vi "BIAS_Client.vi"() -> ()   [LabVIEW 2012]
uses:
  <userlib>/bias2/subvis/ROI_rect.ctl
  <userlib>/bias2/subvis/Imaging_State.ctl
  <userlib>/bias2/subvis/Frame_Controls.ctl
  <userlib>/bias2/subvis/ui/CameraParameters.ctl
  <vilib>/Utility/error.llb/DialogType.ctl
  <userlib>/bias2/classes/CameraBase/CameraBase.lvclass
  <vilib>/event_ctls.llb/lveventtype.ctl
  <userlib>/bias2/subvis/zlock/ZLock.lvclass
  <userlib>/bias2/subvis/ExposureSettings.ctl
  <vilib>/addons/h5labview/H5F_mode.ctl
  <vilib>/Utility/file.llb/Read From Spreadsheet File (DBL).vi
  <vilib>/addons/h5labview/H5File.lvlib
  <vilib>/addons/h5labview/H5GroupObject.lvlib
  <vilib>/addons/h5labview/H5Attrib.lvlib
  <vilib>/addons/h5labview/H5Base.lvlib
  <vilib>/Analysis/NI_AALPro.lvlib
panel:
  in  "capture":T1 caption="Capture"
  in  "tools_zoom":T2 caption="Zoom tools"
  in  "tools_view":cluster{"sel":bool, "in":bool, "out":bool} caption="View tools"
  in  "files":T3 caption="Files"
  in  "stop":bool
  out "stop_time":dbl=11.582550000000003
  out "busy":bool caption="Busy"
  out "recent_error":bool caption="Error"
  out "remote":bool caption="Remote"
  out "acquiring":bool caption="Acquiring"
  out "img_OD":T4(plugin-control)
  out "image_raw":sgl[][](array[numeric])
  in  "tabs":T5(tab)=enum."Internal"
  in  "binning":cluster{"x":u8, "y":u8}={"x"=1, "y"=1}
  in  "effective_pixel":dbl caption="effective pixel size"
  in  "rotation":u16(ring) items=["Do not rotate", "Rotate 90°", "Rotate 180°", "Rotate -90°"]
  out "cam_params":cluster{"String":string, "value":variant}[](array[cluster])=[{"String"="TriggerSource", "value"=variant(string "Freerun")}, {"String"="Timeout", "value"=variant(u32 23583)}, {"String"="ShiftPixelBits", "value"=variant(bool FALSE)}, {"String"="PixelFormat", "value"=variant(string "Mono14")}] caption="Camera Parameters"
  in  "rois":T7(array[cluster])=[{"get"=FALSE, "set"=FALSE, "rect"={"left"=0, "top"=0, "right"=0, "bottom"=0}, "color"=16777224}, {"get"=FALSE, "set"=FALSE, "rect"={"left"=0, "top"=0, "right"=0, "bottom"=0}, "color"=6618880}, {"get"=FALSE, "set"=FALSE, "rect"={"left"=0, "top"=0, "right"=0, "bottom"=0}, "color"=16776960}, {"get"=FALSE, "set"=FALSE, "rect"={"left"=0, "top"=0, "right"=0, "bottom"=0}, "color"=4849919}]
  in  "camera name":string
  out "camera model":string="GX1920 (02-2410B), serial 0xF3101FDAB"
  in  "exposure":sgl=100.0 caption="exposure (ms)"
  out "location":string caption="camera location"
  out "roi_sensor":T6={"left"=0, "top"=0, "right"=1936, "bottom"=1456} caption="camera size"
  out "roi_capture":T6={"left"=686, "top"=399, "right"=1281, "bottom"=1004}
  out "keep":u8
  out "working dir":path
  out "current file":string
  in  "raw_ctrls":T8={"col_scheme"=0, "val_min"=100.0, "val_max"=16384.0, "automax"=FALSE} {"col_scheme" items=["Grayscale", "Rainbow", "Temperature", "-", "AlpineColors", "Amherst", "Aquamarine", "ArmyColors", "AtlanticColors", "AuroraColors", "AvocadoColors", "BeachColors", "BlueGreenYellow", "BrassTones", "BrightBands", "BrownCyanTones", "CandyColors", "CherryTones", "CMYKColors", "CoffeeTones", "DarkBands", "DarkRainbow", "DarkTerrain", "DeepSeaColors", "Default", "FallColors", "FruitPunchColors", "FuchsiaTones", "GrayTones", "GrayYellowTones", "GreenBrownTerrain", "GreenPinkTones", "IslandColors", "LabVIEW", "LakeColors", "LightTemperatureMap", "LightTerrain", "MintColors", "NeonColors", "NIST", "Pastel", "PearlColors", "PigeonTones", "PlumColors", "Rainbow", "RedBlueTones", "RedGreenSplit", "RoseColors", "RustTones", "SandyTerrain", "SiennaTones", "SolarColors", "SouthwestColors", "StarryNightColors", "SunsetColors", "TemperatureMap", "ThermometerColors", "ValentineTones", "WatermelonColors"]; "val_max" format="%_4g"; "val_min" format="%_4g"}
  in  "raw_list":i32(listbox)=-1 caption="Raw Frames"
  in  "hold_frames":bool caption="Hold last flat/dark frames"
  in  "histograms":bool caption="histogram"
  out "recent":string[](array[string]) caption="recent log messages"
  out "state":T9 caption="system state"
  in  "last error":T10={"status"=FALSE, "code"=42, "description"="", "time"=timestamp(3029490000.67111 s since 1904-01-01)} caption="most recent error:" {"time" format="%<%H:%M:%S %d/%m/%y>T"}
  in  "Parameters":T11={"name"="XY_1_Flea3", "sdk"="IMAQdx_Flea3_Firewire", "serial"=0, "port"=1024, "h5"=path "C:/Experiments/rb_chip/connectiontable.h5", "zlock server"="atomchip-1.nist.gov", "zlock port"=7339}
  out "sequencer":T12(array[cluster])
  out "roi_current":T6
  out "image_data":u16[][][](array[numeric])
  out "frame":i32=-1 caption="display_frame"
  out "BLACS port":u16
  out "image_size":i32[](array[numeric])
  out "attribs":variant[](array[variant])=[variant(i32 864), variant(i32 519), variant(i32 1176), variant(i32 878), variant(i64 0), variant(string "Freerun"), variant(u32 1), variant(u32 1), variant(i64 864), variant(i64 519), variant(i64 312), variant(i64 359), variant(dbl 100000.00149011612)]
  out "raw histograms":T13(array[cluster])
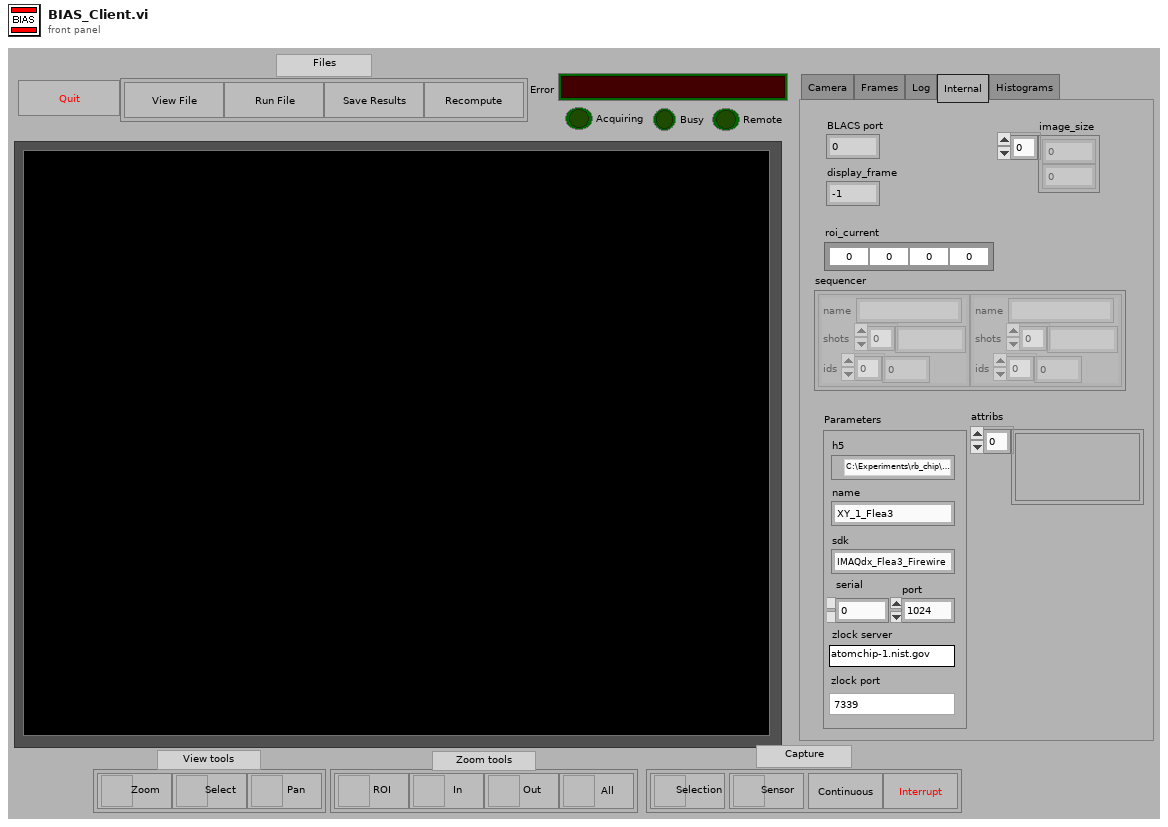
[diagram p1: front panel]
types:
  T1 = cluster{"roi":bool, "chip":bool, "continuous":bool, "abort":bool}
  T2 = cluster{"sel":bool, "in":bool, "out":bool, "all":bool}
  T3 = cluster{"open_file 2":bool, "open_file":bool, "save_file":bool, "open_file 3":bool}
  T4 = typedef "IMAQ Image.ctl" = refnum<image>
  T5 = enum32{"Camera", "Frames", "Log", "Internal", "Histograms"}
  T6 = typedef "ROI_rect.ctl" = cluster{"left":i32, "top":i32, "right":i32, "bottom":i32}
  T7 = cluster{"get":bool, "set":bool, "rect":T6, "color":u32}[]
  T8 = typedef "Frame_Controls.ctl" = cluster{"col_scheme":u16, "val_min":sgl, "val_max":sgl, "automax":bool}
  T9 = typedef "Imaging_State.ctl" = enum16{"<NULL>", "Init", "Read File", "Save File", "Idle", "Compute", "Redraw", "Draw Overlays", "Software trigger", "Acquire", "Fit", "Clear", "Quit"}
  T10 = cluster{"status":bool, "code":i32, "description":string, "time":timestamp}
  T11 = typedef "CameraParameters.ctl" = cluster{"name":string, "sdk":string, "serial":u64, "port":u16, "h5":path, "zlock server":string, "zlock port":u32}
  T12 = cluster{"name":string, "shots":string[], "ids":i32[]}[]
  T13 = cluster{"XY Graph":cluster{"X Values":dbl[], "Histogram: h(x)":i32[]}}[]
  T14 = typedef "DialogType.ctl" = u16
  T15 = typedef "ExposureSettings.ctl" = cluster{"exposure":dbl, "external":bool, "roi":T6, "frames":i32, "binning":cluster{"x":u8, "y":u8}}
  T16 = typedef "H5File.lvlib/H5F_mode.ctl" = enum16{"read-only", "read-write", "overwrite", "create new", "open or create"}
  T17 = typedef "Image Type" = u32
  T18 = cluster{"sensor_width":u16, "sensor_width":u16, "sensor_width":u16, "sensor_height":u16}
  T19 = cluster{"X Values":dbl[], "Histogram: h(x)":i32[]}
  T20 = cluster{"Histogram Graph":cluster{"X Values":dbl[], "Histogram: h(x)":i32[]}}
  T21 = cluster{"name":string, "shots":string[], i32[]}[]
  T22 = typedef "lveventtype.ctl" = enum32{"Null", "Timeout", "Annotation Menu Selection", "Annotation Menu Selection?", "App Instance Close", "App Instance Close?", "Autoscale Range Change", "Cell Edit", "Cell Edit?", "Cursor Grab", "Cursor Grab?", "Cursor Menu Selection", "Cursor Menu Selection?", "Cursor Move", "Cursor Release", "Data Change", "Direction Change", "Display State Change", "Drag Ended", "Drag Enter", "Drag Leave", "Drag Over", "Drag Source Update", "Drag Starting", "Drag Starting?", "Drop", "Exec State Change", "Key Down", "Key Down?", "Key Repeat", "Key Repeat?", "Key Up", "Listbox Double Click", "Menu Activation?", "Menu Selection (App)", "Menu Selection? (App)", "Menu Selection (User)", "Mouse Down", "Mouse Down?", "Mouse Enter", "Mouse Leave", "Mouse Move", "Mouse Up", "NI Security User Change (App)", "Pane Size", "Panel Close", "Panel Close?", "Panel Resize", "Plot Attribute Change", "Scale Range Change", "Shortcut Menu Activation?", "Shortcut Menu Selection (App)", "Shortcut Menu Selection? (App)", "Shortcut Menu Selection (User)", "Tree Double Click", "Tree Drag", "Tree Drag?", "Tree Drop", "Tree Drop?", "Tree Item Close", "Tree Item Close?", "Tree Item Open", "Tree Item Open?", "Value Change"}
  T23 = cluster{"Global Rectangle":i32[], "Contours":cluster{"Contour Type":u32, "ROI Type":u32, "Points":i32[]}[]}
  T24 = typedef "ROI Descriptor" = cluster{"Global Rectangle":i32[], "Contours":cluster{"ID":enum32{"External", "Internal"}, "Type":u32, "Coordinates":i32[]}[]}
  T25 = cluster{"Contour Type":u32, "ROI Type":u32, "Points":i32[]}[]
  T26 = cluster{"FinalVal[0]":bool, "FinalVal[1]":bool, "FinalVal[2]":bool}
  T27 = cluster{"all rows[0]":dbl, "all rows[1]":dbl, "all rows[2]":dbl}
  T28 = cluster{"get":bool, "set":bool, "rect":T6, "color":u32}
  T29 = cluster{"Value":u8, "Value":u8, "Value":u8, "Value":u8}
  T30 = cluster{"col_scheme":u16, "val_min":sgl, "val_max":sgl, "automax":bool}
  T31 = enum16{"Standard", "Buffered", "CRLF", "Immediate"}
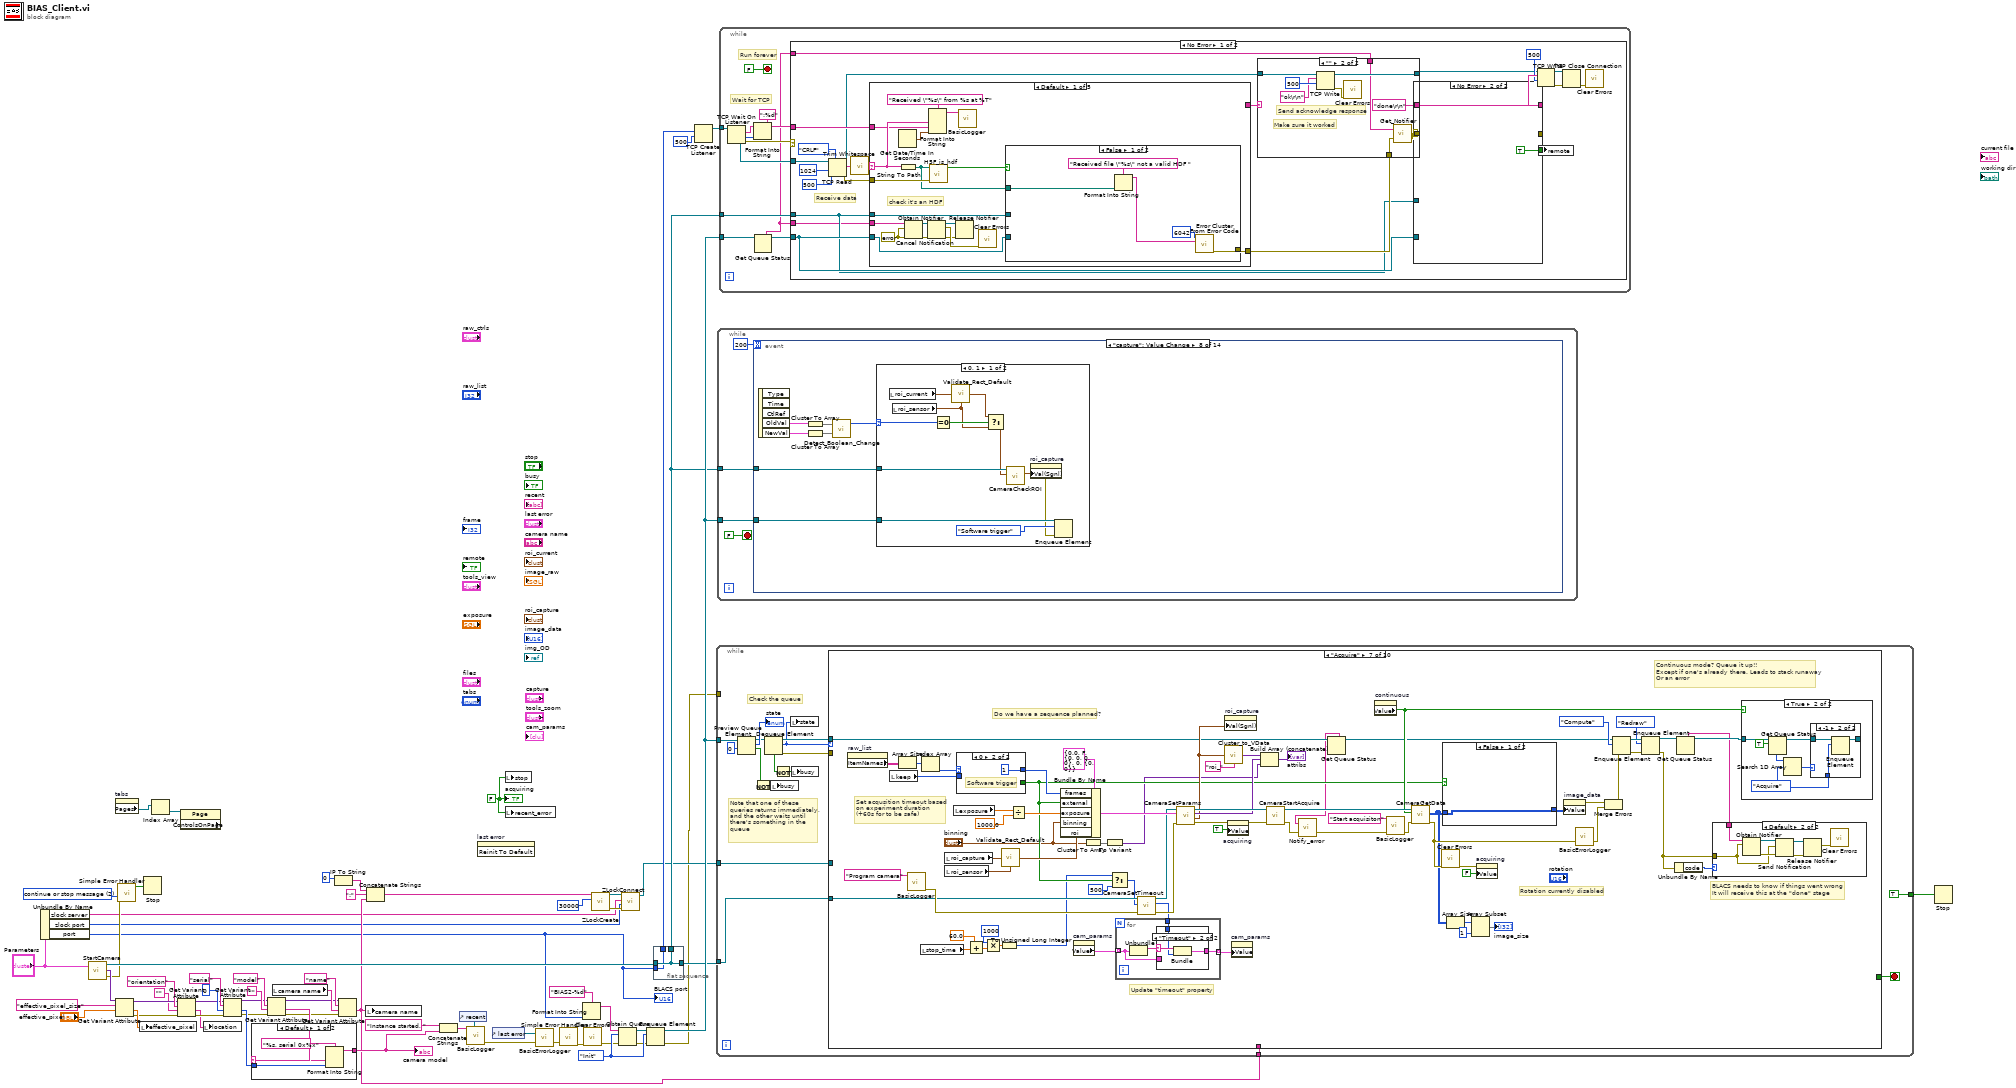
[diagram p0: block diagram]
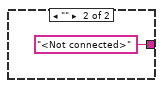
[diagram p2: hidden frame]
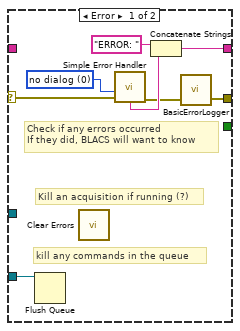
[diagram p3: hidden frame]
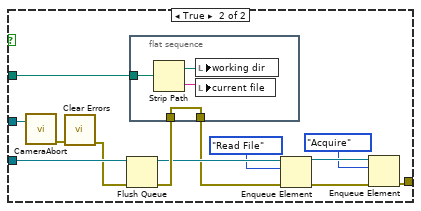
[diagram p5: hidden frame]
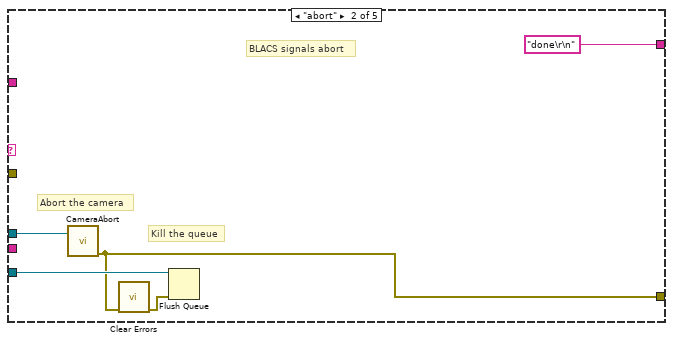
[diagram p6: hidden frame]
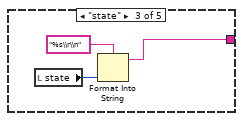
[diagram p7: hidden frame]
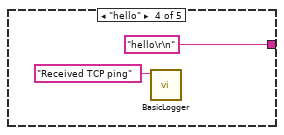
[diagram p8: hidden frame]
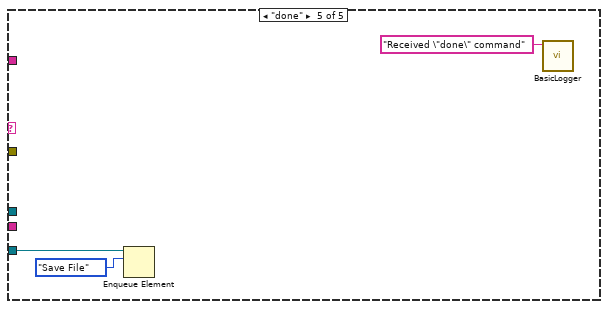
[diagram p9: hidden frame]
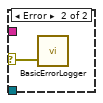
[diagram p10: hidden frame]
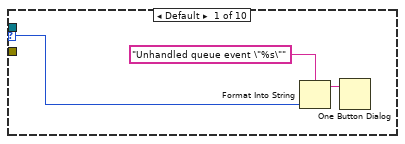
[diagram p11: hidden frame]
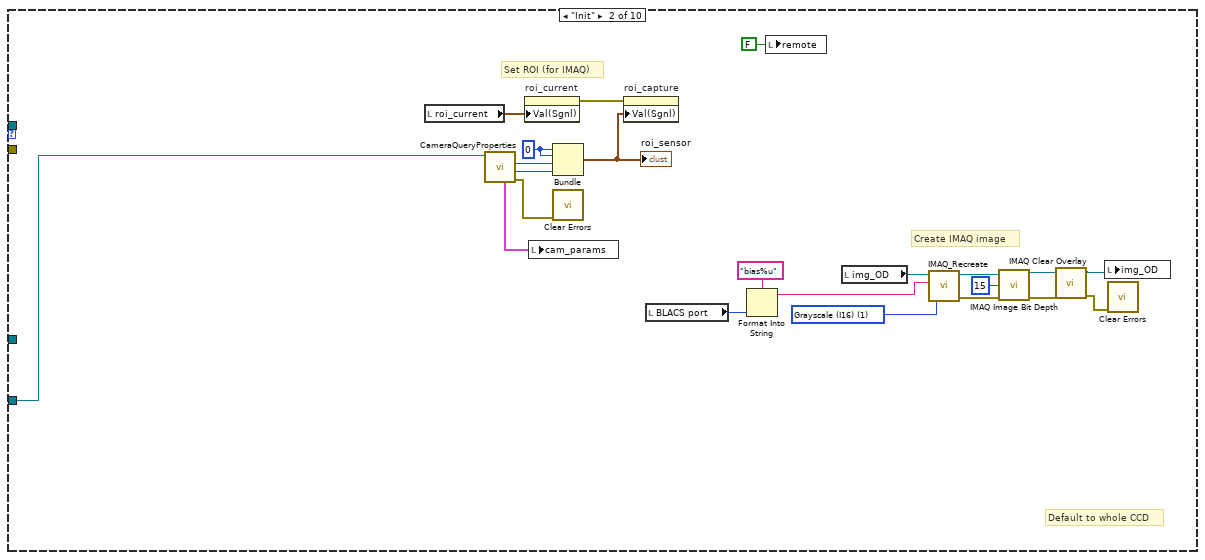
[diagram p12: hidden frame]
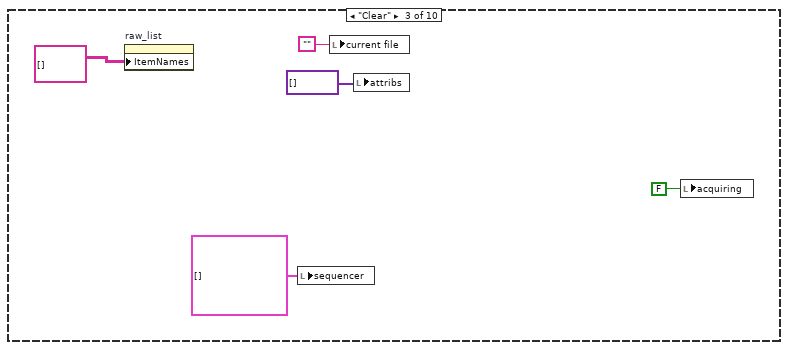
[diagram p13: hidden frame]
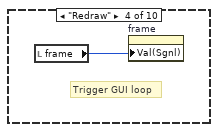
[diagram p14: hidden frame]
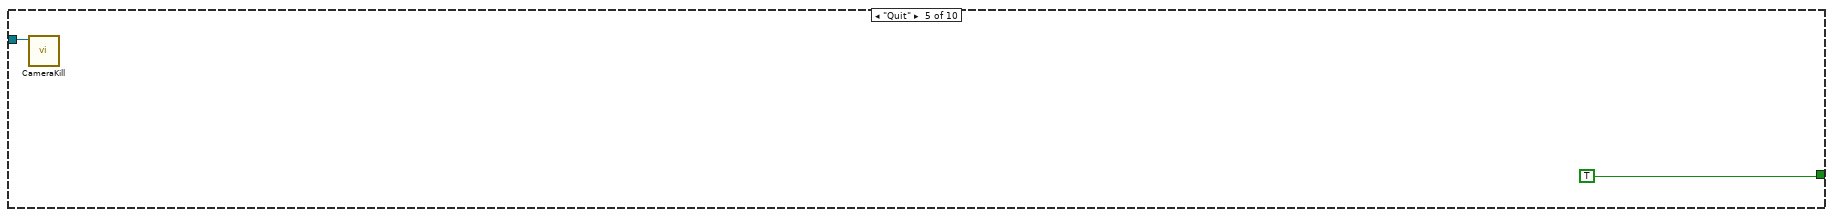
[diagram p15: hidden frame]
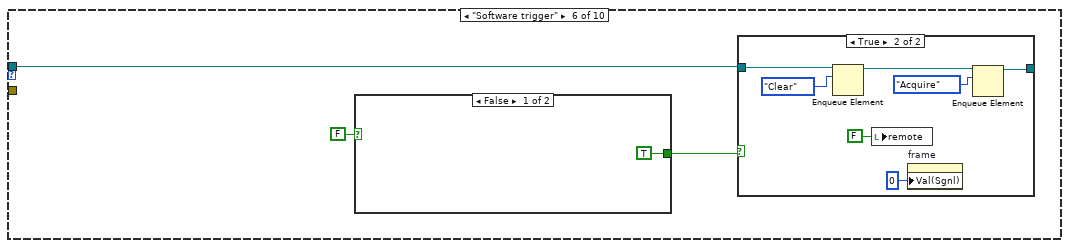
[diagram p16: hidden frame]
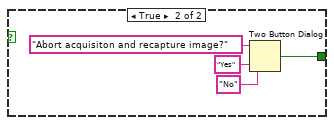
[diagram p18: hidden frame]
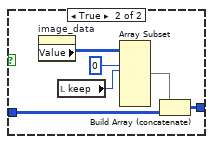
[diagram p19: hidden frame]
diagram:
  w17 = T14 2 items=["no dialog", "OK message", "continue or stop message", "OK message + warnings", "continue/stop + warnings"] ("type of dialog (OK msg:1)")
  w33 = FALSE ("acquiring")
  w64 = Imaging_State."Init" ("Imaging_State")
  n1 = Unbundle By Name("Parameters") -> ("zlock server"=w2:string, "zlock port"=w1:u32, "port"=w5:u16)
  "BLACS port" <- w5
  n2 = call <userlib>:"StartCamera.vi"("Parameters"="Parameters") -> ("camera"=w31:refnum<class "CameraBase.lvclass">, "params"=w40:variant, "error out"=w19:errorcluster)  [unwired: 1 in]
  n3 = property on="tabs" class="TabCtl (strict)"() -> ("Pages"=w8:refnum<vi>[])  [unwired: 2 in, 2 out]
  n4 = Get Variant Attribute(Variant=w40, name="effective_pixel_size", default value (empty Variant)="effective_pixel") -> (duplicate Variant=w25:variant, value=w53:dbl, error out=w22:errorcluster)  [unwired: 1 in, 1 out]
  n5 = call <vilib>:"Simple Error Handler.vi"("type of dialog (OK msg:1)"=w17, "error in (no error)"=w19) -> ("error?"=w18:bool)  [unwired: 3 in, 4 out]
  n6 = local write "effective_pixel"(w53) -> ()
  n7 = Stop(stop? (T)=w18) -> ()
  n8 = Index Array(array=w8) -> (element=w7:refnum<vi>)  [unwired: 1 in]
  n9 = Get Variant Attribute(Variant=w25, name="orientation", default value (empty Variant)="", error in=w22) -> (duplicate Variant=w24:variant, value=w20:string, error out=w21:errorcluster)  [unwired: 1 out]
  n10 = property class="Page" props=["ControlsOnPage"](reference=w7) -> ()  [unwired: 1 in, 3 out]
  n11 = local write "location"(w20) -> ()
  n12 = Get Variant Attribute(Variant=w24, name="serial", default value (empty Variant)=u64 0, error in=w21) -> (duplicate Variant=w37:variant, value=w39:u64, error out=w36:errorcluster)  [unwired: 1 out]
  n13 = Get Variant Attribute(Variant=w37, name="model", default value (empty Variant)="", error in=w36) -> (duplicate Variant=w35:variant, value=w38:string, error out=w34:errorcluster)  [unwired: 1 out]
  n14 = case shown="Default" w38 {
    selector: w38 -> [w66 _]
    tunnel: [w68 "<Not connected>"] -> w42
    tunnel: w39 -> [w67 _]
    frame Default {
      n15 = Format Into String(format string="%s, serial 0x%x", w66, w67) -> (resulting string=w68:string)  [unwired: 2 in, 1 out]
    }
    frame "" {
    }
  }
  "camera model" <- w42
  n16 = local read "camera name"() -> (w41:string)
  n17 = IP To String(2:u32 0 ("net address")) -> (0:w11:string)  [unwired: 1 in]
  n18 = Get Variant Attribute(Variant=w35, name="name", default value (empty Variant)=w41, error in=w34) -> (value=w6:string)  [unwired: 3 out]
  n19 = local write "camera name"(w6) -> ()
  n20 = Concatenate Strings(w11, ":" ("string"), w6) -> (w12:string)
  n21 = Concatenate Strings("Instance started, " ("string"), w42) -> (w43:string)
  n22 = control-ref of="recent"() -> (w45:refnum<vi>)
  n23 = call <userlib>:"BasicLogger.vi"("indicator"=w45, "text"=w43) -> ("error out"=w50:errorcluster)  [unwired: 5 in, 1 out]
  n24 = invoke on="last error" class="Clust (strict)" method="Reinit To Default"() -> ()  [unwired: 3 in, 3 out]
  n25 = control-ref of="last error"() -> (w58:refnum<vi>)
  n26 = local write "stop"(w33) -> ()
  n27 = local write "recent_error"(w33) -> ()
  n28 = call <userlib>:"BasicErrorLogger.vi"("error in"=w50, "indicator"=w58) -> ("error out"=w57:errorcluster)  [unwired: 1 out]
  n29 = call <vilib>:"Simple Error Handler.vi"("error in (no error)"=w57) -> ("error out"=w56:errorcluster)  [unwired: 4 in, 4 out]
  n30 = Format Into String(format string="BIAS2-%d" ("name (unnamed)"), w5) -> (resulting string=w27:string)  [unwired: 2 in, 1 out]
  n31 = call <vilib>:"Clear Errors.vi"("error in (no error)"=w56) -> ("error out"=w55:errorcluster)  [unwired: 6 in]
  n32 = call <userlib>:"ZLockCreate.vi"("timeout (500ms)"=30000 ("reply timeout (500ms)"), "app name"=w12) -> ("error out"=w14:errorcluster, "ZLock out"=w15:refnum<class "ZLock.lvclass">)  [unwired: 4 in]
  n33 = Obtain Queue(name (unnamed)=w27, element data type=w64, error in (no error)=w55) -> (queue out=w65:refnum<queue>, error out=w63:errorcluster)  [unwired: 2 in, 1 out]
  n34 = call-dynamic "ZLockConnect.vi"("error in (no error)"=w14, "port (7339)"=w1, "host"=w2, "ZLock in"=w15) -> ("ZLock out"=w13:refnum<class "ZLock.lvclass">)  [unwired: 6 in, 1 out]
  n35 = Enqueue Element(queue=w65, element=w64, error in (no error)=w63) -> (queue out=w60:refnum<queue>, error out=w3:errorcluster)  [unwired: 1 in, 1 out]
  n36 = flat-sequence {
    tunnel: w5 -> [w71]
    tunnel: w31 -> [w72]
    tunnel: [w72] -> w29
    tunnel: [w72] -> w30
    tunnel: [w71] -> w28
    frame #0 {
    }
  }
  n37 = TCP Create Listener(9:500 ("timeout ms (25000)"), 10:w28) -> (3:w59:refnum<k5>)  [unwired: 3 in, 2 out]
  n38 = while {
    tunnel: [TRUE] -> w62
    tunnel: w30 -> [w84]
    tunnel: w60 -> [w78]
    tunnel: w13 -> [w74]
    tunnel: w3 -> [_]
    tunnel: w6 -> [w73]
    stop <- w85 stop-if-true
    # "Check the queue"
    # "Note that one of these\nqueries returns immediately,\nand the other waits until\nthere's something in the\nqueue"
    n39 = Preview Queue Element(queue=w78, timeout in ms (-1)=0) -> (queue out=w77:refnum<queue>, element=→"state":T9, timed out?=w75:bool)  [unwired: 1 in, 1 out]
    n40 = Not(x=w75) -> (.not. x?=w76:bool)
    n41 = Dequeue Element(queue=w77) -> (queue out=w88:refnum<queue>, element=w83:T9, timed out?=w82:bool, error out=w87:errorcluster)  [unwired: 2 in]
    n42 = local write "busy"(w76) -> ()
    n43 = Not(x=w82) -> (.not. x?=w81:bool)
    n44 = local write "state"(w83) -> ()
    n45 = local write "busy"(w81) -> ()
    n46 = case shown="\"Acquire\"" w83 {
      selector: w83 -> [w90 _ _ _ _ _ _ _ _ _]
      tunnel: w88 -> [_ _ _ _ _ w123 w140 _ w264 w393]
      tunnel: w87 -> [_ _ _ _ _ _ _ _ _ _]
      tunnel: [_ _ _ _ TRUE _ _ _ _ _] -> w85
      tunnel: w84 -> [_ w97 _ _ w120 _ w179 _ _ _]
      tunnel: w74 -> [_ _ _ _ _ _ _ _ w259 w394]
      tunnel: w73 -> [_ _ _ _ _ _ _ _ _ _]
      frame Default {
        n47 = Format Into String(format string="Unhandled queue event \"%s\"", w90) -> (resulting string=w89:string)  [unwired: 2 in, 1 out]
        n48 = One Button Dialog(message=w89) -> ()  [unwired: 1 in, 1 out]
      }
      frame "Init" {
        w96 = u16 0 ("sensor_width")
        w112 = T17 1 items=["Grayscale (U8)", "Grayscale (I16)", "Grayscale (SGL)", "Complex (CSG)", "RGB (U32)", "HSL (U32)", "RGB (U64)", "Grayscale (U16)"] ("type")
        # "Create IMAQ image"
        # "Default to whole CCD"
        # "Set ROI (for IMAQ)"
        n49 = local read "roi_current"() -> (w107:T6)
        n50 = call-dynamic "CameraQueryProperties.vi"("CameraBase in"=w97) -> ("error out"=w98:errorcluster, "sensor_height"=w106:u16, "sensor_width"=w105:u16, "cam_params"=w104:cluster{"String":string, "value":variant}[])  [unwired: 6 in, 1 out]
        n51 = property on="roi_current" class="Clust (strict)"("Val(Sgnl)"=w107) -> (error out=w108:errorcluster)  [unwired: 2 in, 1 out]
        n52 = local write "cam_params"(w104) -> ()
        n53 = Bundle("sensor_width"=w96, "sensor_width"=w96, "sensor_width"=w105, "sensor_height"=w106) -> (w95:T18)  [unwired: 1 in]
        "roi_sensor" <- w95
        n54 = call <vilib>:"Clear Errors.vi"("error in (no error)"=w98) -> ()  [unwired: 6 in, 1 out]
        n55 = property on="roi_capture" class="Clust (strict)"(error in=w108, "Val(Sgnl)"=w95) -> ()  [unwired: 1 in, 2 out]
        n56 = local read "BLACS port"() -> (w94:u16)
        n57 = Format Into String(format string="bias%u", w94) -> (resulting string=w92:string)  [unwired: 2 in, 1 out]
        n58 = local write "remote"(FALSE ("remote")) -> ()
        n59 = local read "img_OD"() -> (w113:T4)
        n60 = call <userlib>:"IMAQ_Recreate.vi"("type"=w112, "name"=w92, "image in"=w113) -> ("error out"=w109:errorcluster, "image out"=w111:T4)  [unwired: 3 in]
        n61 = call "IMAQ Image Bit Depth"("Image"=w111, "Bit Depth (0)"=u32 15, "error in (no error)"=w109) -> ("Image Out"=w102:T4, "error out"=w103:errorcluster)  [unwired: 10 in, 1 out]
        n62 = call "IMAQ Clear Overlay"("error in (no error)"=w103, "Image"=w102) -> ("error out"=w100:errorcluster, "Image Out"=w101:T4)  [unwired: 8 in]
        n63 = local write "img_OD"(w101) -> ()
        n64 = call <vilib>:"Clear Errors.vi"("error in (no error)"=w100) -> ()  [unwired: 6 in, 1 out]
      }
      frame "Clear" {
        n65 = property on="raw_list" class="MCListbox (strict)"("ItemNames"=string[][] [] ("sequence")) -> ()  [unwired: 2 in, 2 out]
        n66 = local write "sequencer"(T12 [] ("sequencer")) -> ()
        n67 = local write "current file"("") -> ()
        n68 = local write "attribs"(variant[] []) -> ()
        n69 = local write "acquiring"(FALSE ("pending")) -> ()
      }
      frame "Redraw" {
        # "Trigger GUI loop"
        n70 = local read "frame"() -> (w119:i32)
        n71 = property on="frame" class="DigNum (strict)"("Val(Sgnl)"=w119) -> ()  [unwired: 2 in, 2 out]
      }
      frame "Quit" {
        n72 = call-dynamic "CameraKill.vi"("CameraBase in"=w120) -> ()  [unwired: 9 in, 2 out]
      }
      frame "Software trigger" {
        n73 = case shown="False" FALSE {
          tunnel: [TRUE ("T button?") w134] -> w124
          frame False {
          }
          frame True {
            n74 = Two Button Dialog(message="Abort acquisiton and recapture image?", 1:"No" ("F button name (\"Cancel\")"), 2:"Yes" ("T button name (\"OK\")")) -> (T button?=w134:bool)
          }
        }
        n75 = case shown="True" w124 {
          tunnel: [w125 w131] -> _
          tunnel: w123 -> [w125 w130]
          frame False {
          }
          frame True {
            n76 = Enqueue Element(queue=w130, element=Imaging_State."Clear") -> (queue out=w129:refnum<queue>)  [unwired: 2 in, 2 out]
            n77 = local write "remote"(FALSE ("remote")) -> ()
            n78 = property on="frame" class="DigNum (strict)"("Val(Sgnl)"=0 ("Value (Signaling)")) -> ()  [unwired: 2 in, 2 out]
            n79 = Enqueue Element(queue=w129, element=Imaging_State."Acquire") -> (queue out=w131:refnum<queue>)  [unwired: 2 in, 2 out]
          }
        }
      }
      frame "Acquire" {
        # "Update \"timeout\" property"
        # "Rotation currently disabled"
        # "Set acqusition timeout based\non experiment duration\n(+60s for to be safe)"
        # "BLACS needs to know if things went wrong\nIt will receive this at the \"done\" stage"
        # "Continuous mode? Queue it up!!\nExcept if one's already there. Leads to stack runaway\nOr an error"
        # "Do we have a sequence planned?"
        n80 = property on="raw_list" class="MCListbox (strict)"() -> ("ItemNames"=w190:string[][])  [unwired: 2 in, 2 out]
        n81 = local read "keep"() -> (w183:u8)
        n82 = Array Size(array=w190) -> (size(s)=w189:i32[])
        n83 = call <userlib>:"BasicLogger.vi"("text"="Program camera") -> ("error out"=w180:errorcluster)  [unwired: 6 in, 1 out]
        n84 = local read "stop_time"() -> (w174:dbl)
        n85 = Index Array(array=w189) -> (element=w188:i32)  [unwired: 1 in]
        n86 = local read "roi_capture"() -> (w204:T6)
        n87 = local read "roi_sensor"() -> (w199:T6)
        n88 = local read "exposure"() -> (w208:sgl)
        n89 = case shown="0" w188 {
          selector: w188 -> [w242 _]
          tunnel: [w243 1] -> w163
          tunnel: [TRUE ("external") _] -> w154
          tunnel: w183 -> [w241 _]
          frame Default {
            n90 = Subtract(x=w242, y=w241) -> (x-y=w243:i32)
          }
          frame 0 {
            # "Software trigger"
          }
        }
        n91 = Add(x=60.0, y=w174) -> (x+y=w175:dbl)
        n92 = Multiply(x=u32 1000 ("col"), y=w175) -> (x*y=w182:dbl)
        n93 = To Unsigned Long Integer(number=w182) -> (unsigned 32bit integer=w153:u32)
        n94 = call <userlib>:"Validate_Rect_Default.vi"("rect"=w204, "default"=w199) -> ("out"=w167:T6)
        n95 = Divide(x=w208, y=sgl 1000.0) -> (x/y=w203:sgl)
        n96 = Bundle By Name(cluster=T15 {"exposure"=0.0, "external"=FALSE, "roi"={"left"=0, "top"=0, "right"=0, "bottom"=0}, "frames"=0, "binning"={"x"=0, "y"=0}} ("settings"), "frames"=w163, "external"=w154, "exposure"=w203, "binning"="binning", "roi"=w167) -> (w202:T15)
        n97 = property on="cam_params" class="Arr (strict)"() -> ("Value"=w162:cluster{"String":string, "value":variant}[])  [unwired: 2 in, 2 out]
        n98 = Cluster To Array(cluster="binning") -> (array=w144:u8[])
        n99 = To Variant(anything=w144) -> (Variant=w145:variant)
        n100 = Select(t=w153, s=w154, f=u32 500) -> (s? t:f=w152:u32)
        n101 = call-dynamic "CameraSetTimeout.vi"("error in (no error)"=w180, "Timeout"=w152, "CameraBase in"=w179) -> ("error out"=w178:errorcluster, "Timeout set"=w176:u32, "CameraBase out"=w177:refnum<class "CameraBase.lvclass">)  [unwired: 6 in]
        n102 = for {
          tunnel: w162 -> [w216] mode=indexing
          tunnel: w176 -> [w217]
          tunnel: [w219] -> w161 mode=indexing
          n103 = Unbundle(w216) -> ("String"=w218:string)  [unwired: 1 out]
          n104 = case shown="\"Timeout\"" w218 {
            selector: w218 -> [_ w222]
            tunnel: [w220 w223] -> w219
            tunnel: w217 -> [_ w221]
            tunnel: w216 -> [w220 _]
            frame Default {
            }
            frame "Timeout" {
              n105 = Bundle(w222, "Timeout set"=w221) -> (w223:cluster{string, "Timeout set":u32})  [unwired: 1 in]
            }
          }
        }
        n106 = call-dynamic "CameraSetParams.vi"("error in (no error)"=w178, "settings"=w202, "CameraBase in"=w177) -> ("error out"=w195:errorcluster, "roi_out"=w170:T6, "attributes"=w187:variant[], "CameraBase out"=w194:refnum<class "CameraBase.lvclass">)  [unwired: 5 in]
        n107 = call <userlib>:"Cluster_to_VData.vi"("cluster"=w170, "prefix"="roi_") -> ("vdata"=w186:variant[])
        n108 = property on="roi_capture" class="Clust (strict)"("Val(Sgnl)"=w170) -> ()  [unwired: 2 in, 2 out]
        n109 = property on="acquiring" class="Bool (strict)"(error in=w195, "Value"=TRUE ("acquiring")) -> (error out=w192:errorcluster)  [unwired: 1 in, 1 out]
        n110 = property on="cam_params" class="Arr (strict)"("Value"=w161) -> ()  [unwired: 2 in, 2 out]
        n111 = Build Array (concatenate)(w186, w187, w145) -> (→"attribs":variant[])
        n112 = call-dynamic "CameraStartAcquire.vi"("error in (no error)"=w192, "CameraBase in"=w194) -> ("error out"=w172:errorcluster, "CameraBase out"=w193:refnum<class "CameraBase.lvclass">)  [unwired: 8 in]
        n113 = Get Queue Status(queue=w140) -> (queue out=w139:refnum<queue>, queue name=w138:string)  [unwired: 2 in, 6 out]
        n114 = call <userlib>:"Notify_error.vi"("error in"=w172, "name"=w138) -> ("error out"=w169:errorcluster)  [unwired: 1 in]
        n115 = property on="continuous" class="Bool (strict)"() -> ("Value"=w166:bool)  [unwired: 2 in, 2 out]
        n116 = call <userlib>:"BasicLogger.vi"("error in"=w169, "text"="Start acquisiton") -> ("error out"=w191:errorcluster)  [unwired: 5 in, 1 out]
        n117 = call-dynamic "CameraGetData.vi"("error in (no error)"=w191, "keep open?"=w166, "CameraBase in"=w193) -> ("error out"=w206:errorcluster, "image_data"=w150:u16[][][])  [unwired: 6 in, 1 out]
        n118 = call <vilib>:"Clear Errors.vi"("error in (no error)"=w206) -> ("error out"=w196:errorcluster)  [unwired: 6 in]
        n119 = case shown="False" w154 {
          tunnel: [w209 w212] -> w171
          tunnel: w150 -> [w209 w210]
          frame False {
          }
          frame True {
            n120 = property on="image_data" class="Arr (strict)"() -> ("Value"=w211:u16[][][])  [unwired: 2 in, 2 out]
            n121 = local read "keep"() -> (w214:u8)
            n122 = Array Subset(array=w211, index (dim 0)=0 ("index"), length (dim 0)=w214) -> (w213:u16[][][])  [unwired: 4 in]
            n123 = Build Array (concatenate)(w213, w210) -> (w212:u16[][][])
          }
        }
        n124 = Array Size(array=w150) -> (size(s)=w149:i32[])
        n125 = Array Subset(array=w149, index=1) -> (→"image_size":i32[])  [unwired: 1 in]
        n126 = property on="acquiring" class="Bool (strict)"(error in=w196, "Value"=FALSE ("acquiring")) -> ()  [unwired: 1 in, 2 out]
        n127 = property on="image_data" class="Arr (strict)"("Value"=w171) -> (error out=w165:errorcluster)  [unwired: 2 in, 1 out]
        n128 = call <userlib>:"BasicErrorLogger.vi"("error in"=w206) -> ("error out"=w164:errorcluster)  [unwired: 1 in, 1 out]
        n129 = Merge Errors(w165, w164) -> (w157:errorcluster)
        n130 = Enqueue Element(queue=w139, element=Imaging_State."Compute", error in (no error)=w157) -> (queue out=w160:refnum<queue>, error out=w156:errorcluster)  [unwired: 1 in, 1 out]
        n131 = Enqueue Element(queue=w160, element=Imaging_State."Redraw", error in (no error)=w156) -> (queue out=w143:refnum<queue>, error out=w155:errorcluster)  [unwired: 1 in, 1 out]
        n132 = Unbundle By Name(w155) -> ("code"=w184:i32)
        n133 = Get Queue Status(queue=w143) -> (queue out=w142:refnum<queue>, queue name=w141:string)  [unwired: 2 in, 6 out]
        n134 = case shown="Default" w184 {
          tunnel: w155 -> [_ w225]
          tunnel: w141 -> [_ w224]
          frame 0, 5024 {
            # "Fine or Abort"
          }
          frame Default {
            n135 = Obtain Notifier(name (unnamed)=w224, notification data type=w225) -> (notifier out=w227:refnum<notifier>, error out=w228:errorcluster)  [unwired: 2 in, 1 out]
            n136 = Send Notification(notification=w225, notifier=w227, error in (no error)=w228) -> (notifier out=w230:refnum<notifier>, error out=w229:errorcluster)
            n137 = Release Notifier(notifier=w230, error in (no error)=w229) -> (last notification=w226:errorcluster)  [unwired: 1 in, 2 out]
            n138 = call <vilib>:"Clear Errors.vi"("error in (no error)"=w226) -> ()  [unwired: 6 in, 1 out]
          }
        }
        n139 = case shown="True" w166 {
          tunnel: w142 -> [_ w236]
          frame False {
          }
          frame True {
            w231 = Imaging_State."Acquire" ("element")
            n140 = Get Queue Status(queue=w236, return elements? (F)=TRUE) -> (queue out=w232:refnum<queue>, elements=w234:T9[])  [unwired: 1 in, 6 out]
            n141 = Search 1D Array(1D array=w234, element=w231) -> (index of element=w233:i32)  [unwired: 1 in]
            n142 = case shown="-1" w233 {
              tunnel: [w237 w240] -> _
              tunnel: w232 -> [w237 w239]
              tunnel: w231 -> [_ w238]
              frame Default {
              }
              frame -1 {
                n143 = Enqueue Element(queue=w239, element=w238) -> (queue out=w240:refnum<queue>)  [unwired: 2 in, 2 out]
              }
            }
          }
        }
      }
      frame "Compute" {
        n144 = case shown="True" "histograms" {
          frame False {
          }
          frame True {
            # "Raw image histograms (very slow)"
            n145 = property on="image_data" class="Arr (strict)"() -> ("Value"=w248:u16[][][])  [unwired: 2 in, 2 out]
            n146 = for {
              tunnel: w248 -> [w256] mode=indexing
              tunnel: [w252] -> w249 mode=indexing
              n147 = Array Size(array=w256) -> (size(s)=w258:i32[])
              n148 = Multiply Array Elements(1:w258) -> (0:w257:i32)
              n149 = Reshape Array(w256, w257) -> (w255:u16[])
              n150 = call <vilib>:"General Histogram.vi"("X"=w255, "max"=16384.0, "min"=0.0, "# bins"=400 ("intervals")) -> ("Histogram Graph"=w253:T19)  [unwired: 7 in, 4 out]
              n151 = Bundle("Histogram Graph"=w253) -> (w252:T20)  [unwired: 1 in]
            }
            "raw histograms" <- w249
          }
        }
        n152 = local read "frame"() -> (w246:i32)
        n153 = property on="frame" class="DigNum (strict)"("Val(Sgnl)"=w246) -> ()  [unwired: 2 in, 2 out]
      }
      frame "Read File" {
        n154 = local write "recent_error"(FALSE ("recent_error")) -> ()
        n155 = local read "working dir"() -> (w263:path)
        n156 = local read "current file"() -> (w262:string)
        n157 = property on="continuous" class="Bool (strict)"("Value"=FALSE ("continuous")) -> ()  [unwired: 2 in, 2 out]
        n158 = case shown="Default" w262 {
          selector: w262 -> [w291 _]
          tunnel: w264 -> [w297 _]
          tunnel: w263 -> [w292 _]
          tunnel: w259 -> [w274 _]
          tunnel: [w267 _] -> _
          frame Default {
            n159 = local read "camera name"() -> (w294:string)
            n160 = Build Path(base path=w292, name or relative path=w291) -> (appended path=w275:path)
            n161 = Path To String(path=w275) -> (string=w276:string)
            n162 = call-dynamic "ZLockAcquire.vi"("key"=w276, "ZLock in"=w274) -> ("error out"=w268:errorcluster, "key out"=w272:string, "ZLock out"=w273:refnum<class "ZLock.lvclass">)  [unwired: 7 in]
            n163 = Concatenate Strings("Read file  " ("text"), w291) -> (w296:string)
            n164 = call <vilib>:"H5F_open.vi"("error in (no error)"=w268, "mode"=H5F_mode."read-only", "path"=w275) -> ("error out"=w284:errorcluster, "ref"=w281:i32)  [unwired: 1 in]
            n165 = Concatenate Strings("/devices/" ("Name"), w294) -> (w280:string)
            n166 = call <userlib>:"BasicLogger.vi"("text"=w296) -> ()  [unwired: 6 in, 2 out]
            n167 = call <vilib>:"H5G_open.vi"("error in (no error)"=w284, "name"=w280, "ref"=w281) -> ("error out"=w283:errorcluster, "group"=w282:i32)  [unwired: 3 in]
            n168 = case shown="No Error" w283 {
              selector: w283 -> [_ w380]
              tunnel: [w347 w379] -> w288
              tunnel: w282 -> [w325 _]
              tunnel: [w345 w382] -> w289
              tunnel: [w334 w378] -> w287
              tunnel: [w341 w383] -> w286
              tunnel: w281 -> [w338 w382]
              frame No Error {
                w352 = "EXPOSURES" ("name")
                # "When is the experiment scheduled to finish?"
                n169 = call <vilib>:"H5A_read_dbl.vi"("attrib_name"="exposure_time" ("attribute"), "ref"=w325) -> ("error out"=w322:errorcluster, "ref out"=w324:i32, "value"=w320:dbl)  [unwired: 5 in]
                n170 = Multiply(x=w320, y=1000.0) -> (x*y=w348:dbl)
                n171 = local write "exposure"(w348) -> ()
                n172 = call <vilib>:"H5A_read_str.vi"("attrib_name"="orientation" ("attribute"), "error in (no error)"=w322, "ref"=w324) -> ("error out"=w318:errorcluster, "ref out"=w350:i32, "value"=w319:string)  [unwired: 4 in]
                "location" <- w319
                n173 = Concatenate Strings("/images/" ("Name"), w319) -> (w339:string)
                n174 = call <vilib>:"H5D_read_col_str.vi"("column"=u16 2, "error in (no error)"=w318, "table"=w352, "ref"=w350) -> ("error out"=w331:errorcluster, "ref out"=w353:i32, "data"=w330:string[])  [unwired: 2 in, 1 out]
                n175 = call <vilib>:"H5D_read_col_str.vi"("column"=u16 0, "error in (no error)"=w331, "table"=w352, "ref"=w353) -> ("error out"=w332:errorcluster, "ref out"=w349:i32, "data"=w328:string[])  [unwired: 2 in, 1 out]
                n176 = call <vilib>:"H5A_read_dbl.vi"("attrib_name"="stop_time" ("attribute"), "obj_name"="/devices/pulseblaster_0" ("Name"), "ref"=w338) -> ("error out"=w316:errorcluster, "ref out"=w345:i32, "value"=w317:dbl)  [unwired: 4 in]
                n177 = call <vilib>:"H5G_close.vi"("error in (no error)"=w332, "ref"=w349) -> ("error out"=w344:errorcluster)  [unwired: 3 in]
                n178 = case shown="No Error" w316 {
                  tunnel: w317 -> [w377 _]
                  frame No Error {
                    "stop_time" <- w377
                  }
                  frame Error {
                  }
                }
                n179 = call <vilib>:"H5L_exists.vi"("path"=w339, "loc_id"=w338) -> ("path out"=w333:string, "exists?"=w340:bool, "loc_id out"=w337:i32)  [unwired: 1 in, 1 out]
                n180 = property on="image_data" class="Arr (strict)"() -> ("Value"=w327:u16[][][])  [unwired: 2 in, 2 out]
                n181 = property on="raw_list" class="MCListbox (strict)"() -> ("ItemNames"=w343:string[][])  [unwired: 2 in, 2 out]
                n182 = call <userlib>:"Fix Sequence.vi"("sequences"=w328, "shots"=w330, "old sequence list"=w343, "image_data"=w327, "keep?"="hold_frames") -> ("sequencer"=w341:T21, "held data"=w336:u16[][][])
                n183 = case shown="True" w340 {
                  tunnel: [w356 w376] -> w347
                  tunnel: w333 -> [_ w375]
                  tunnel: [_ w374] -> w335
                  tunnel: w337 -> [_ w368]
                  tunnel: w344 -> [w356 w367]
                  tunnel: w341 -> [_ w366]
                  frame False {
                    # "Group doesn't exist yet, this is a new shot"
                  }
                  frame True {
                    w358 = u8[] [1, 1]
                    # "Expect attribs\nto exist"
                    n184 = call <vilib>:"H5G_open.vi"("error in (no error)"=w367, "name"=w375, "ref"=w368) -> ("error out"=w364:errorcluster, "group"=w365:i32)  [unwired: 3 in]
                    n185 = call <vilib>:"H5A_read_var.vi"("attrib_name"="binning", "error in (no error)"=w364, "default"=w358, "ref"=w365) -> ("error out"=w361:errorcluster, "ref out"=w362:i32, "value"=w360:variant)  [unwired: 3 in]
                    n186 = Variant To Data(type=w358, Variant=w360) -> (data=w359:u8[])  [unwired: 1 in, 1 out]
                    n187 = local read "roi_capture"() -> (w370:T6)
                    n188 = Array To Cluster(array=w359) -> (cluster=w357:cluster{"[0]":u8, "[1]":u8})
                    n189 = call <userlib>:"Read_Exposures.vi"("ref in"=w362, "sequencer"=w366, "error in"=w361) -> ("ref out"=w372:i32, "ROI"=w371:T6, "loaded images"=w374:u16[][][], "error out"=w373:errorcluster)  [unwired: 1 in, 1 out]
                    n190 = local write "binning"(w357) -> ()
                    n191 = call <userlib>:"Validate_Rect_Default.vi"("rect"=w371, "default"=w370) -> ("out"=w369:T6)
                    n192 = local write "roi_capture"(w369) -> ()
                    n193 = call <vilib>:"H5G_close.vi"("error in (no error)"=w373, "ref"=w372) -> ("error out"=w376:errorcluster)  [unwired: 3 in]
                  }
                }
                n194 = Build Array (concatenate)(w336, w335) -> (w334:u16[][][])
              }
              frame Error {
                n195 = Greater Than 0?(x=w382) -> (x > 0?=w381:bool)
                n196 = case shown="True" w381 {
                  tunnel: w380 -> [w385 _]
                  tunnel: [w385 w388] -> w379
                  frame False {
                  }
                  frame True {
                    n197 = local read "camera name"() -> (w386:string)
                    n198 = Concatenate Strings("Specified HDF has no instructions for camera " ("error message (\"\")"), w386) -> (w387:string)
                    n199 = call <vilib>:"Error Cluster From Error Code.vi"("error message (\"\")"=w387, "error code (0)"=6013) -> ("error out"=w388:errorcluster)  [unwired: 7 in]
                  }
                }
                n200 = local write "current file"("") -> ()
                n201 = local read "sequencer"() -> (w383:T12)
                n202 = property on="image_data" class="Arr (strict)"() -> ("Value"=w378:u16[][][])  [unwired: 2 in, 2 out]
              }
            }
            "sequencer" <- w286
            n203 = Get Queue Status(queue=w297) -> (queue out=w266:refnum<queue>, queue name=w265:string)  [unwired: 2 in, 6 out]
            n204 = call <vilib>:"H5F_close.vi"("error in (no error)"=w288, "ref"=w289) -> ("error out"=w270:errorcluster)  [unwired: 3 in]
            n205 = local write "image_data"(w287) -> ()
            n206 = case shown="Error" w270 {
              selector: w270 -> [_ w312]
              tunnel: [w310 w315] -> _
              tunnel: w266 -> [w310 w314]
              tunnel: w265 -> [_ w311]
              frame No Error {
              }
              frame Error {
                n207 = call <userlib>:"Notify_error.vi"("error in"=w312, "name"=w311) -> ()  [unwired: 1 in, 1 out]
                n208 = local write "current file"("") -> ()
                n209 = Flush Queue(queue=w314) -> (queue out=w315:refnum<queue>)  [unwired: 1 in, 2 out]
              }
            }
            n210 = for {
              tunnel: w286 -> [w306] mode=indexing
              tunnel: [w303] -> w285 mode=indexing
              shift-right: [w300] -> w279
              shift-left: string[][] [] -> [w299]
              n211 = Unbundle(w306) -> ("name"=w301:string, "shots"=w302:string[])  [unwired: 1 out]
              n212 = Equal?(x=w301, y="(held)") -> (x = y?=w304:bool)
              n213 = for {
                tunnel: w302 -> [w309] mode=indexing
                tunnel: w301 -> [w308]
                tunnel: [w307] -> w298 mode=indexing
                n214 = Build Array(w308, w309) -> (w307:string[])
              }
              n215 = Boolean To (0,1)(Boolean=w304) -> (0, 1=w303:i16)
              n216 = Build Array (concatenate)(w298, w299) -> (w300:string[][])
            }
            n217 = call <vilib>:"Clear Errors.vi"("error in (no error)"=w270) -> ("error out"=w271:errorcluster)  [unwired: 6 in]
            n218 = Merge Errors(w268, w271) -> (w269:errorcluster)
            n219 = call-dynamic "ZLockRelease.vi"("error in (no error)"=w269, "key"=w272, "ZLock in"=w273) -> ("error out"=w267:errorcluster)  [unwired: 6 in, 2 out]
            n220 = Add Array Elements(numeric array=w285) -> (sum=→"keep":i16)
            n221 = property on="raw_list" class="MCListbox (strict)"("ItemNames"=w279) -> ()  [unwired: 2 in, 2 out]
          }
          frame "" {
            n222 = call <userlib>:"BasicLogger.vi"("text"="Empty \"read file\" command") -> ()  [unwired: 6 in, 2 out]
          }
        }
      }
      frame "Save File" {
        n223 = local read "working dir"() -> (w397:path)
        n224 = local read "current file"() -> (w396:string)
        n225 = Get Queue Status(queue=w393) -> (queue name=w392:string)  [unwired: 2 in, 7 out]
        n226 = case shown="Default" w396 {
          selector: w396 -> [w416 _]
          tunnel: w397 -> [w417 _]
          tunnel: [w405 w464] -> w395
          tunnel: w394 -> [w402 _]
          tunnel: [w400 _] -> _
          frame Default {
            n227 = Build Path(base path=w417, name or relative path=w416) -> (appended path=w407:path)
            n228 = Path To String(path=w407) -> (string=w406:string)
            n229 = local read "location"() -> (w419:string)
            n230 = call-dynamic "ZLockAcquire.vi"("key"=w406, "ZLock in"=w402) -> ("error out"=w398:errorcluster, "key out"=w403:string, "ZLock out"=w401:refnum<class "ZLock.lvclass">)  [unwired: 7 in]
            n231 = Concatenate Strings("Save file  " ("text"), w416) -> (w420:string)
            n232 = call <vilib>:"H5F_open.vi"("error in (no error)"=w398, "mode"=H5F_mode."read-write", "path"=w407) -> ("error out"=w414:errorcluster, "ref"=w408:i32)  [unwired: 1 in]
            n233 = Concatenate Strings("images/" ("attribute"), w419) -> (w412:string)
            n234 = call <userlib>:"BasicLogger.vi"("text"=w420) -> ()  [unwired: 6 in, 2 out]
            n235 = call <vilib>:"H5G_open.vi"("error in (no error)"=w414, "create? (F)"=TRUE, "name"=w412, "ref"=w408) -> ("error out"=w413:errorcluster, "group"=w410:i32)  [unwired: 2 in]
            n236 = case shown="No Error" w413 {
              selector: w413 -> [_ w461]
              tunnel: [w428 w461] -> w409
              tunnel: w410 -> [w427 _]
              frame No Error {
                n237 = property on="rois" class="Arr (strict)"() -> ("Value"=w426:T7)  [unwired: 2 in, 2 out]
                n238 = local read "effective_pixel"() -> (w436:dbl)
                n239 = local read "camera name"() -> (w440:string)
                n240 = for {
                  tunnel: w427 -> [w451]
                  tunnel: w426 -> [w443] mode=indexing
                  tunnel: [w449] -> w425
                  shift-right: [w448] -> w424
                  shift-left: _ -> [w447]
                  i -> [w446]
                  n241 = Unbundle(w443) -> ("rect"=w442:T6)  [unwired: 3 out]
                  n242 = Format Into String(format string="roi%d", w446) -> (resulting string=w444:string)  [unwired: 2 in, 1 out]
                  n243 = call <userlib>:"Validate_Rect.vi"("rect"=w442) -> ("valid"=w441:bool)
                  n244 = case shown="True" w441 {
                    tunnel: w451 -> [w453 w460]
                    tunnel: TRUE ("overwrite? (F)") -> [_ w459]
                    tunnel: [w453 w458] -> w449
                    tunnel: [w452 w457] -> w448
                    tunnel: w447 -> [w452 w456]
                    tunnel: w444 -> [_ w455]
                    tunnel: w442 -> [_ w454]
                    frame False {
                    }
                    frame True {
                      n245 = call <vilib>:"H5A_write.vi"("value"=w454, "attrib_name"=w455, "error in (no error)"=w456, "overwrite? (F)"=w459, "ref"=w460) -> ("error out"=w457:errorcluster, "ref out"=w458:i32)  [unwired: 3 in]
                    }
                  }
                }
                n246 = local read "attribs"() -> (w438:variant[])
                n247 = call <userlib>:"Set Data Name__ogtk.vi"("Data Name"="effective_pixel_size", "Data"=w436) -> ("Renamed Data"=w434:variant)  [unwired: 8 in, 1 out]
                n248 = call <userlib>:"Set Data Name__ogtk.vi"("Data Name"="camera", "Data"=w440) -> ("Renamed Data"=w437:variant)  [unwired: 8 in, 1 out]
                n249 = Build Array (concatenate)(w434, w438, w437) -> (w433:variant[])
                n250 = property on="image_data" class="Arr (strict)"() -> ("Value"=w423:u16[][][])  [unwired: 2 in, 2 out]
                n251 = call <vilib>:"H5A_write_multi.vi"("attribs"=w433, "overwrite?"=FALSE, "ref"=w425) -> ("error out"=w429:errorcluster, "ref out"=w431:i32)  [unwired: 5 in]
                n252 = property on="sequencer" class="Arr (strict)"() -> ("Value"=w422:T12)  [unwired: 2 in, 2 out]
                n253 = call <vilib>:"Clear Errors.vi"("error in (no error)"=w429) -> ()  [unwired: 6 in, 1 out]
                n254 = call <userlib>:"Write_raw_data.vi"("image_data"=w423, "sequencer"=w422, "ref in"=w431) -> ("error out"=w430:errorcluster)  [unwired: 3 in, 1 out]
                n255 = Merge Errors(w430, w424) -> (w428:errorcluster)
              }
              frame Error {
              }
            }
            n256 = call <vilib>:"H5F_close.vi"("error in (no error)"=w409, "ref"=w408) -> ("error out"=w405:errorcluster)  [unwired: 3 in]
            n257 = call <vilib>:"Clear Errors.vi"("error in (no error)"=w405) -> ("error out"=w404:errorcluster)  [unwired: 6 in]
            n258 = Merge Errors(w398, w404) -> (w399:errorcluster)
            n259 = call-dynamic "ZLockRelease.vi"("error in (no error)"=w399, "key"=w403, "ZLock in"=w401) -> ("error out"=w400:errorcluster)  [unwired: 6 in, 2 out]
          }
          frame "" {
            n260 = call <vilib>:"Error Cluster From Error Code.vi"("error message (\"\")"="Cannot save file - no filename specified" ("error message (\"\")"), "error code (0)"=6015) -> ("error out"=w464:errorcluster)  [unwired: 7 in]
          }
        }
        n261 = call <userlib>:"Notify_error.vi"("error in"=w395, "name"=w392) -> ()  [unwired: 1 in, 1 out]
      }
    }
  }
  n262 = while {
    tunnel: w29 -> [w466]
    tunnel: w60 -> [w467]
    stop <- FALSE stop-if-true
    n263 = event shown="[7] \"capture\": Value Change" {
      selector: _ -> [_ _ _ _ _ _ _ _ _ _ _ _ _ _]
      dyn-events: _ -> [_ _ _ _ _ _ _ _ _ _ _ _ _ _]
      timeout: 200 -> [_ _ _ _ _ _ _ _ _ _ _ _ _ _]
      tunnel: w467 -> [_ _ w489 w492 w535 _ _ w605 _ _ _ _ _ _]
      tunnel: w466 -> [w469 _ _ _ w534 _ _ w604 _ _ _ _ _ _]
      event Timeout {
        w471 = 4 items=["None", "Selection Tool", "Point Tool", "Line Tool", "Rectangle Tool", "Oval Tool", "Polygon Tool", "ClosedFreehandTool", "Annulus Tool", "Rotated Rectangle Tool", "Zoom Tool", "Pan Tool", "Polyline Tool", "Freehand Tool"] ("Tool")
        n264 = event-data() -> ()  [unwired: 1 in, 2 out]
        n265 = invoke on="img_OD" class="ImageControl" method="Get Last Event"("Which Events"=i32[] [2, 1]) -> ("Tool"=w472:i32)  [unwired: 7 in, 7 out]
        n266 = Equal?(x=w472, y=w471) -> (x = y?=w470:bool)
        n267 = case shown="False" w470 {
          tunnel: w469 -> [_ _]
          frame False {
          }
          frame True {
            n268 = local read "binning"() -> (w474:cluster{"x":u8, "y":u8})
            n269 = property on="img_OD" class="ImageControl"() -> ("ROI"=w480:T23)  [unwired: 2 in, 2 out]
            n270 = call <userlib>:"ROI_to_rects.vi"("binning"=w474, "ROI"=w480) -> ("rect"=w479:T6)  [unwired: 3 out]
            n271 = local read "roi_capture"() -> (w478:T6)
            n272 = local read "roi_capture"() -> (w476:T6)
            n273 = call <userlib>:"Apply_Rect_Offset.vi"("offset rect"=w478, "input"=w479) -> ("output"=w477:T6)  [unwired: 3 in]
            n274 = call <userlib>:"Clip_Rect.vi"("bounds"=w476, "rect"=w477) -> ("result"=w475:T6)  [unwired: 1 in]
            n275 = property on="roi_current" class="Clust (strict)"("Val(Sgnl)"=w475) -> ()  [unwired: 2 in, 2 out]
          }
        }
      }
      event Value Change {
        # "Something with interrupts to improve flicker"
        n276 = event-data() -> ()  [unwired: 1 in, 5 out]
        n277 = local read "roi_capture"() -> (w486:T6)
        n278 = local read "roi_current"() -> (w482:T6)
        n279 = Negate(x=w486) -> (-x=w485:T6)
        n280 = local read "binning"() -> (w481:cluster{"x":u8, "y":u8})
        n281 = call <userlib>:"Apply_Rect_Offset.vi"("offset rect"=w485, "input"=w482) -> ("output"=w484:T6)  [unwired: 3 in]
        n282 = call <userlib>:"Rect_to_ROI.vi"("rect"=w484, "binning"=w481) -> ("ROI"=w483:T24)
        n283 = property on="img_OD" class="ImageControl"("ROI"=w483) -> ()  [unwired: 2 in, 2 out]
      }
      event "stop": Value Change {
        n284 = event-data() -> ()  [unwired: 1 in, 5 out]
        n285 = Flush Queue(queue=w489) -> (queue out=w487:refnum<queue>)  [unwired: 1 in, 2 out]
        n286 = Enqueue Element(queue=w487, element=Imaging_State."Quit") -> ()  [unwired: 2 in, 3 out]
      }
      event "files": Value Change {
        n287 = event-data() -> ("OldVal"=w494:T3, "NewVal"=w493:T3)  [unwired: 1 in, 3 out]
        n288 = Cluster To Array(cluster=w494) -> (array=w496:bool[])
        n289 = Cluster To Array(cluster=w493) -> (array=w495:bool[])
        n290 = call <userlib>:"Detect_Boolean_Change.vi"("NewVal"=w495, "OldVal"=w496) -> ("ButtonId"=w491:i32)  [unwired: 2 out]
        n291 = Greater Or Equal To 0?(x=w491) -> (x >= 0?=w490:bool)
        n292 = case shown="True" w490 {
          tunnel: w492 -> [_ w497]
          tunnel: w491 -> [_ w498]
          frame False {
          }
          frame True {
            n293 = local read "current file"() -> (w499:string)
            n294 = case shown="0, 1" w498 {
              selector: w498 -> [_ _ _ w506]
              tunnel: w499 -> [_ _ _ w514]
              tunnel: w497 -> [w500 w502 _ w507]
              frame 2 {
                n295 = Enqueue Element(queue=w500, element=Imaging_State."Save File") -> ()  [unwired: 2 in, 3 out]
              }
              frame 3 {
                n296 = Enqueue Element(queue=w502, element=Imaging_State."Compute") -> ()  [unwired: 2 in, 3 out]
              }
              frame Default {
              }
              frame 0, 1 {
                n297 = local read "working dir"() -> (w511:path)
                n298 = call "File Dialog"("start path"=w511, "prompt"="Select H5 File", "default name"=w514, "pattern (all files)"="*.h5", "pattern label"="HDF files") -> ("selected path"=w512:path, "error out"=w505:errorcluster)  [unwired: 7 in, 2 out]
                n299 = call <vilib>:"H5F_is_hdf.vi"("error in (no error)"=w505, "path"=w512) -> ("error out"=w504:errorcluster, "valid"=w513:bool)  [unwired: 1 in, 1 out]
                n300 = case shown="False" w513 {
                  tunnel: w512 -> [_ w527]
                  tunnel: w507 -> [_ w526]
                  tunnel: w506 -> [_ w516]
                  tunnel: w504 -> [_ _]
                  frame False {
                    n301 = One Button Dialog(message="Chosen file is not a valid HDF5") -> ()  [unwired: 1 in, 1 out]
                  }
                  frame True {
                    n302 = Flush Queue(queue=w526) -> (queue out=w522:refnum<queue>, remaining elements=w525:T9[])  [unwired: 1 in, 1 out]
                    n303 = Strip Path(path=w527) -> (stripped path=w524:path, name=w523:string)
                    n304 = property on="working dir" class="Path"("Value"=w524) -> (error out=w519:errorcluster)  [unwired: 2 in, 1 out]
                    n305 = Array Size(array=w525) -> (size(s)=w517:i32)
                    n306 = property on="current file" class="Str"(error in=w519, "Value"=w523) -> (error out=w518:errorcluster)  [unwired: 1 in, 1 out]
                    n307 = Enqueue Element(queue=w522, element=Imaging_State."Read File", error in (no error)=w518) -> (queue out=w520:refnum<queue>)  [unwired: 1 in, 2 out]
                    n308 = case shown="Default" w517 {
                      frame 0 {
                      }
                      frame Default {
                        n309 = call <userlib>:"BasicLogger.vi"("text"="File open forced queue clear") -> ()  [unwired: 6 in, 2 out]
                      }
                    }
                    n310 = case shown="Default" w516 {
                      tunnel: w520 -> [w530 w531]
                      frame Default {
                        n311 = Enqueue Element(queue=w530, element=Imaging_State."Redraw") -> ()  [unwired: 2 in, 3 out]
                      }
                      frame 1 {
                        n312 = Enqueue Element(queue=w531, element=Imaging_State."Acquire") -> ()  [unwired: 2 in, 3 out]
                      }
                    }
                  }
                }
              }
            }
          }
        }
      }
      event "capture.abort": Value Change {
        n313 = event-data() -> ("NewVal"=w533:bool)  [unwired: 1 in, 4 out]
        n314 = case shown="True" w533 {
          tunnel: w535 -> [_ w540]
          tunnel: w534 -> [_ w539]
          tunnel: [_ w536] -> _
          frame False {
          }
          frame True {
            n315 = Flush Queue(queue=w540) -> (error out=w537:errorcluster)  [unwired: 1 in, 2 out]
            n316 = call-dynamic "CameraAbort.vi"("error in (no error)"=w537, "CameraBase in"=w539) -> ("error out"=w536:errorcluster)  [unwired: 8 in, 1 out]
            n317 = call <userlib>:"BasicLogger.vi"("text"="Abort signalled") -> ()  [unwired: 6 in, 2 out]
          }
        }
      }
      event "tools_zoom": Value Change {
        n318 = event-data() -> ("OldVal"=w544:T2, "NewVal"=w543:T2)  [unwired: 1 in, 3 out]
        n319 = control-ref of="img_OD"() -> (w541:refnum<vi>)
        n320 = Cluster To Array(cluster=w544) -> (array=w545:bool[])
        n321 = Cluster To Array(cluster=w543) -> (array=w546:bool[])
        n322 = call <userlib>:"Detect_Boolean_Change.vi"("NewVal"=w546, "OldVal"=w545) -> ("ButtonId"=w547:i32)  [unwired: 2 out]
        n323 = Build Array(w541) -> (w542:refnum<vi>[])
        n324 = for {
          tunnel: w547 -> [w549]
          tunnel: [w548] -> _ mode=indexing
          tunnel: w542 -> [w548] mode=indexing
          n325 = case shown="1" w549 {
            tunnel: w548 -> [w550 w568 w580 w588 _]
            frame 0 {
              n326 = property on="Property Node" class="ImageControl" props=["ROI", "Image Area Size", "Image Area Height", "Image Area Width"](reference=w550) -> (reference out=w551:refnum<vi>, "ROI"=w557:T23, "Image Area Height"=w556:u32, "Image Area Width"=w555:u32)  [unwired: 1 in, 2 out]
              n327 = Unbundle(w557) -> ("Global Rectangle"=w554:i32[], "Contours"=w553:T25)
              n328 = Empty Array?(array=w553) -> (empty?=w552:bool)
              n329 = case shown="False" w552 {
                tunnel: w556 -> [w566 _]
                tunnel: w555 -> [w565 _]
                tunnel: w554 -> [w562 _]
                tunnel: w551 -> [w558 _]
                frame False {
                  n330 = formula code="Zx=W/(R[2]-R[0]);\nZy=H/(R[3]-R[1]);\nCx=(R[2]+R[0])/2;\nCy=(R[3]+R[1])/2;"("R"=w562, "H"=w566, "W"=w565) -> ("Zx"=w560:dbl, "Zy"=w561:dbl, "Cx"=w564:dbl, "Cy"=w563:dbl)
                  n331 = Max & Min(x=w560, y=w561) -> (min(x,y)=w559:dbl)  [unwired: 1 out]
                  n332 = property on="Property Node" class="ImageControl"(reference=w558, "X Zoom"=w559, "Y Zoom"=w559, "Image Center X Position"=w564, "Image Center Y Position"=w563) -> ()  [unwired: 1 in, 2 out]
                }
                frame True {
                }
              }
            }
            frame 1 {
              w575 = sgl 1.2 ("x")
              # "Zoom to ROI if possible"
              n333 = property on="Property Node" class="ImageControl"(reference=w568) -> (reference out=w569:refnum<vi>, "X Zoom"=w576:sgl, "Y Zoom"=w577:sgl, "ROI"=w574:T23, "Image Center Position"=w570:cluster{"X":u32, "Y":u32})  [unwired: 1 in, 1 out]
              n334 = local read "binning"() -> (w567:cluster{"x":u8, "y":u8})
              n335 = call <userlib>:"ROI_to_rects.vi"("binning"=w567, "ROI"=w574) -> ("center"=w572:cluster{"x":i16, "y":i16}, "valid"=w573:bool)  [unwired: 2 out]
              n336 = Select(t=w572, s=w573, f=w570) -> (s? t:f=w571:cluster{"X":u32, "Y":u32})
              n337 = Multiply(x=w576, y=w575) -> (x*y=w579:sgl)
              n338 = Multiply(x=w577, y=w575) -> (x*y=w578:sgl)
              n339 = property on="Property Node" class="ImageControl"(reference=w569, "X Zoom"=w579, "Y Zoom"=w578, "Image Center Position"=w571) -> ()  [unwired: 1 in, 2 out]
            }
            frame 2 {
              w582 = sgl 1.2 ("x")
              n340 = property on="Property Node" class="ImageControl"(reference=w580) -> (reference out=w581:refnum<vi>, "X Zoom"=w584:sgl, "Y Zoom"=w585:sgl, "Image Center Position"=w583:cluster{"X":u32, "Y":u32})  [unwired: 1 in, 1 out]
              n341 = Divide(x=w584, y=w582) -> (x/y=w587:sgl)
              n342 = Divide(x=w585, y=w582) -> (x/y=w586:sgl)
              n343 = property on="Property Node" class="ImageControl"(reference=w581, "X Zoom"=w587, "Y Zoom"=w586, "Image Center Position"=w583) -> ()  [unwired: 1 in, 2 out]
            }
            frame 3 {
              n344 = property on="Property Node" class="ImageControl"(reference=w588, "Zoom to Fit Mode"=TRUE) -> ()  [unwired: 1 in, 2 out]
            }
            frame Default {
            }
          }
        }
      }
      event "tools_view": Value Change {
        n345 = event-data() -> ("OldVal"=w592:cluster{"sel":bool, "in":bool, "out":bool}, "NewVal"=w591:cluster{"sel":bool, "in":bool, "out":bool})  [unwired: 1 in, 3 out]
        n346 = Cluster To Array(cluster=w592) -> (array=w599:bool[])
        n347 = Cluster To Array(cluster=w591) -> (array=w598:bool[])
        n348 = call <userlib>:"Detect_Boolean_Change.vi"("NewVal"=w598, "OldVal"=w599) -> ("FinalVal"=w596:bool[], "SingleEvent"=w594:bool, "ButtonId"=w597:i32)
        n349 = Array To Cluster(array=w596) -> (cluster=w593:T26)
        n350 = Select(t=w593, s=w594, f=w592) -> (s? t:f=w590:cluster{"sel":bool, "in":bool, "out":bool})
        n351 = case shown="0" w597 {
          tunnel: [w600 w601 w602 w603] -> w595
          frame Default {
            n352 = property on="img_OD" class="ImageControl"() -> ("Current ROI Tool"=w600:u32)  [unwired: 2 in, 2 out]
          }
          frame 0 {
            w601 = u32 8 items=["No Selection", "Point", "Line", "Rectangle", "Oval", "Polygon", "Freehand Region", "Annulus", "Zoom", "Pan", "Broken Line", "Freehand Line", "Rotated Rectangle"] ("Tool (Point)")
          }
          frame 1 {
            w602 = u32 3 items=["No Selection", "Point", "Line", "Rectangle", "Oval", "Polygon", "Freehand Region", "Annulus", "Zoom", "Pan", "Broken Line", "Freehand Line", "Rotated Rectangle"] ("Tool (Point)")
          }
          frame 2 {
            w603 = u32 9 items=["No Selection", "Point", "Line", "Rectangle", "Oval", "Polygon", "Freehand Region", "Annulus", "Zoom", "Pan", "Broken Line", "Freehand Line", "Rotated Rectangle"] ("Tool (Point)")
          }
        }
        n353 = local write "tools_view"(w590) -> ()
        n354 = property on="img_OD" class="ImageControl"("Current ROI Tool"=w595) -> ()  [unwired: 2 in, 2 out]
      }
      event "capture": Value Change {
        n355 = event-data() -> ("OldVal"=w606:T1, "NewVal"=w607:T1)  [unwired: 1 in, 3 out]
        n356 = Cluster To Array(cluster=w606) -> (array=w610:bool[])
        n357 = Cluster To Array(cluster=w607) -> (array=w609:bool[])
        n358 = call <userlib>:"Detect_Boolean_Change.vi"("NewVal"=w609, "OldVal"=w610) -> ("ButtonId"=w608:i32)  [unwired: 2 out]
        n359 = case shown="0, 1" w608 {
          selector: w608 -> [w619 _]
          tunnel: w605 -> [w615 _]
          tunnel: w604 -> [w613 _]
          frame 0, 1 {
            n360 = local read "roi_current"() -> (w621:T6)
            n361 = local read "roi_sensor"() -> (w618:T6)
            n362 = Equal To 0?(x=w619) -> (x = 0?=w620:bool)
            n363 = call <userlib>:"Validate_Rect_Default.vi"("rect"=w621, "default"=w618) -> ("out"=w617:T6)
            n364 = Select(t=w617, s=w620, f=w618) -> (s? t:f=w612:T6)
            n365 = call-dynamic "CameraCheckROI.vi"("ROI_in"=w612, "CameraBase in"=w613) -> ("ROI_out"=w611:T6)  [unwired: 7 in, 2 out]
            n366 = property on="roi_capture" class="Clust (strict)"("Val(Sgnl)"=w611) -> (error out=w614:errorcluster)  [unwired: 2 in, 1 out]
            n367 = Enqueue Element(queue=w615, element=Imaging_State."Software trigger", error in (no error)=w614) -> ()  [unwired: 1 in, 3 out]
          }
          frame Default {
          }
        }
      }
      event Value Change {
        # "try to avoid infinite loop"
        n368 = event-data() -> ("CtlRef"=w632:refnum<vi>, "OldVal"=w625:T8, "NewVal"=w624:T8)  [unwired: 1 in, 2 out]
        n369 = Unbundle By Name(w624) -> ("col_scheme"=w628:u16)
        n370 = Unbundle By Name(w625) -> ("col_scheme"=w627:u16)
        n371 = Unbundle By Name(w624) -> ("val_max"=w631:sgl)
        n372 = Unbundle By Name(w625) -> ("val_max"=w630:sgl)
        n373 = Not Equal?(x=w625, y=w624) -> (x != y?=w622:bool)
        n374 = Equal?(x=w628, y=w627) -> (x = y?=w626:bool)
        n375 = Not Equal?(x=w631, y=w630) -> (x != y?=w633:bool)
        n376 = And(x=w622, y=w626) -> (x .and. y?=w623:bool)
        n377 = case shown="True" w633 {
          tunnel: w632 -> [_ w638]
          tunnel: [_ w639] -> w629
          tunnel: w624 -> [_ w636]
          frame False {
          }
          frame True {
            n378 = Bundle By Name(cluster=w636, "automax"=FALSE) -> (w637:T8)
            n379 = property class="Clust (strict)"(reference=w638, "Value"=w637) -> (error out=w639:errorcluster)  [unwired: 1 in, 1 out]
          }
        }
        n380 = case shown="True" w623 {
          tunnel: w629 -> [_ w635]
          frame False {
          }
          frame True {
            n381 = local read "frame"() -> (w634:i32)
            n382 = property on="frame" class="DigNum (strict)"(error in=w635, "Val(Sgnl)"=w634) -> ()  [unwired: 1 in, 2 out]
          }
        }
      }
      event Value Change {
        n383 = event-data() -> ("CtlRef"=w641:refnum<vi>, "NewVal"=w645:u16)  [unwired: 1 in, 3 out]
        n384 = property class="Ring (strict)"(reference=w641) -> ("Owner"=w647:refnum<vi>)  [unwired: 1 in, 2 out]
        n385 = local read "frame"() -> (w648:i32)
        n386 = control-ref of="raw_ctrls"() -> (w646:refnum<vi>)
        n387 = Equal?(x=w647, y=w646) -> (x = y?=w644:bool)
        n388 = Greater Or Equal To 0?(x=w648) -> (x >= 0?=w643:bool)
        n389 = Not Exclusive Or(1:w643, 2:w644) -> (0:w642:bool)
        n390 = case shown="True" w642 {
          tunnel: w645 -> [_ w652]
          tunnel: w641 -> [_ w649]
          frame False {
          }
          frame True {
            n391 = case shown="0" w652 {
              tunnel: [w656 w664 w665 w666 w668] -> w651
              tunnel: [w655 _ _ _ w667] -> w650
              tunnel: w649 -> [w654 _ _ _ _]
              frame Default {
                w656 = u32 5 items=["Grayscale", "Binary", "Gradient", "Rainbow", "Temperature", "User Defined"] ("Palette:Palette Type")
                n392 = property on="Property Node" class="Ring (strict)"(reference=w654) -> ("RingText.Text"=w653:string)  [unwired: 1 in, 2 out]
                n393 = Concatenate Strings(w653, ".tsv" ("string")) -> (w657:string)
                n394 = Build Path(base path=path "Z:/Temp/rgb gradients", name or relative path=w657) -> (appended path=w660:path)
                n395 = call-poly <vilib>:"Read From Spreadsheet File.vi"("file path (dialog if empty)"=w660) -> ("all rows"=w661:dbl[][])  [unwired: 6 in, 4 out]
                n396 = for {
                  tunnel: w661 -> [w663] mode=indexing
                  tunnel: [w662] -> w655 mode=indexing
                  n397 = Array To Cluster(array=w663) -> (cluster=w662:T27)
                }
              }
              frame 0 {
                w664 = u32 0 items=["Grayscale", "Binary", "Gradient", "Rainbow", "Temperature", "User Defined"] ("Palette:Palette Type")
              }
              frame 1 {
                w665 = u32 3 items=["Grayscale", "Binary", "Gradient", "Rainbow", "Temperature", "User Defined"] ("Palette:Palette Type")
              }
              frame 2 {
                w666 = u32 4 items=["Grayscale", "Binary", "Gradient", "Rainbow", "Temperature", "User Defined"] ("Palette:Palette Type")
              }
              frame 3 {
                n398 = property on="img_OD" class="ImageControl"() -> ("Palette Type"=w668:u32, "User Palette"=w667:cluster{"Red":u8, "Green":u8, "Blue":u8}[])  [unwired: 2 in, 2 out]
              }
            }
            n399 = property on="img_OD" class="ImageControl"("Palette Type"=w651, "User Palette"=w650) -> ()  [unwired: 2 in, 2 out]
          }
        }
      }
      event "last error.status": Value Change; "last error.status", "recent_error": Mouse Up {
        n400 = event-data() -> ("Type"=w673:T22, "CtlRef"=w669:refnum<vi>)  [unwired: 1 in, 2 out]
        n401 = Equal?(x=lveventtype."Mouse Up" ("Type"), y=w673) -> (x = y?=w671:bool)
        n402 = case shown="False" w671 {
          tunnel: [w675 FALSE ("recent_error")] -> w670
          tunnel: w669 -> [w674 _]
          frame False {
            n403 = property on="Property Node" class="Bool (strict)"(reference=w674) -> ("Value"=w675:bool)  [unwired: 1 in, 2 out]
          }
          frame True {
          }
        }
        "recent_error" <- w670
      }
      event "raw_list": Value Change {
        n404 = event-data() -> ("CtlRef"=w684:refnum<vi>, "OldVal"=w682:i32, "NewVal"=w683:i32)  [unwired: 1 in, 2 out]
        n405 = Greater Or Equal To 0?(x=w682) -> (x >= 0?=w681:bool)
        n406 = Not Equal?(x=w682, y=w683) -> (x != y?=w686:bool)
        n407 = Greater Or Equal To 0?(x=w683) -> (x >= 0?=w680:bool)
        n408 = And(x=w686, y=w680) -> (x .and. y?=w685:bool)
        n409 = Exclusive Or(1:w681, 2:w680) -> (0:w679:bool)
        n410 = case shown="True" w685 {
          tunnel: w684 -> [_ w696]
          tunnel: w683 -> [_ w695]
          tunnel: w679 -> [_ w691]
          tunnel: [_ w690] -> w678
          tunnel: [w687 w689] -> w677
          frame False {
            n411 = local read "frame"() -> (w687:i32)
          }
          frame True {
            # "Set the other one to -1"
            n412 = control-ref of="raw_list"() -> (w688:refnum<vi>)
            n413 = Equal?(x=w688, y=w696) -> (x = y?=w692:bool)
            n414 = Negate(x=w695) -> (-x=w697:i32)
            n415 = Decrement(x=w697) -> (x-1=w694:i32)
            n416 = Select(t=w695, s=w692, f=w694) -> (s? t:f=w689:i32)
            n417 = case shown="True" w691 {
              frame False {
              }
              frame True {
                n418 = control-ref of="col_scheme"() -> (w698:refnum<vi>)
                n419 = property class="Ring (strict)"(reference=w698) -> (reference out=w701:refnum<vi>, error out=w700:errorcluster, "Value"=w699:u16)  [unwired: 1 in]
                n420 = property class="Ring (strict)"(reference=w701, error in=w700, "Val(Sgnl)"=w699) -> ()  [unwired: 2 out]
              }
            }
            n421 = property class="MCListbox (strict)"(reference=w688, "Value"=-1) -> (error out=w690:errorcluster)  [unwired: 1 in, 1 out]
          }
        }
        n422 = property on="frame" class="DigNum (strict)"(error in=w678, "Val(Sgnl)"=w677) -> ()  [unwired: 1 in, 2 out]
      }
      event "rois": Value Change {
        n423 = event-data() -> ("CtlRef"=w703:refnum<vi>, "NewVal"=w705:T7)  [unwired: 1 in, 3 out]
        n424 = for {
          tunnel: w705 -> [w740] mode=indexing
          tunnel: [w737] -> w704 mode=indexing
          w738 = FALSE ("get")
          n425 = Unbundle(w740) -> ("get"=w745:bool, "set"=w744:bool, "rect"=w741:T6)  [unwired: 1 out]
          n426 = Build Array(w745, w744) -> (w743:bool[])
          n427 = Boolean Array To Number(Boolean array=w743) -> (number=w742:u32)
          n428 = case shown="Default" w742 {
            tunnel: w741 -> [w746 _ w748]
            tunnel: [w746 w747 w748] -> w739
            frame Default {
            }
            frame 1 {
              # "set using roi_current"
              n429 = local read "roi_current"() -> (w747:T6)
            }
            frame 2 {
              n430 = property on="roi_current" class="Clust (strict)"("Val(Sgnl)"=w748) -> ()  [unwired: 2 in, 2 out]
            }
          }
          n431 = Bundle(cluster=w740, "get"=w738, "set"=w738, "rect"=w739) -> (w737:T28)  [unwired: 1 in]
        }
        n432 = property class="Arr (strict)"(reference=w703, "Value"=w704) -> (error out=w702:errorcluster)  [unwired: 1 in, 1 out]
        n433 = flat-sequence {
          tunnel: w702 -> [_]
          frame #0 {
            n434 = local read "img_OD"() -> (w710:T4)
            n435 = call "IMAQ Clear Overlay"("Groups"=string[] ["roi"], "Image"=w710) -> ("error out"=w714:errorcluster, "Image Out"=w712:T4)  [unwired: 8 in]
            n436 = call <vilib>:"Clear Errors.vi"("error in (no error)"=w714) -> ()  [unwired: 6 in, 1 out]
            n437 = local read "roi_capture"() -> (w715:T6)
            n438 = Build Array (concatenate)("rois") -> (w709:T7)
            n439 = Negate(x=w715) -> (-x=w716:T6)
            n440 = property on="x" class="DigNum (strict)"() -> ("Value"=w707:u8)  [unwired: 2 in, 2 out]
            n441 = property on="y" class="DigNum (strict)"() -> ("Value"=w706:u8)  [unwired: 2 in, 2 out]
            n442 = Bundle("Value"=w707, "Value"=w706, "Value"=w707, "Value"=w706) -> (w717:T29)  [unwired: 1 in]
            n443 = for {
              tunnel: w709 -> [w725] mode=indexing
              shift-right: [w722] -> w713
              shift-left: w712 -> [w726]
              tunnel: w716 -> [w719]
              tunnel: w717 -> [w718]
              n444 = Unbundle By Name(w725) -> ("color"=w723:u32, "rect"=w720:T6)
              n445 = Not Equal?(x=u32 16777216, y=w723) -> (x != y?=w721:bool)
              n446 = case shown="True" w721 {
                tunnel: w726 -> [w727 w736]
                tunnel: w723 -> [_ w734]
                tunnel: [w727 w733] -> w722
                tunnel: w720 -> [_ w732]
                tunnel: w719 -> [_ w731]
                tunnel: w718 -> [_ w729]
                frame False {
                }
                frame True {
                  n447 = call <userlib>:"Apply_Rect_Offset.vi"("offset rect"=w731, "input"=w732) -> ("output"=w730:T6)  [unwired: 3 in]
                  n448 = Quotient & Remainder(x=w730, y=w729) -> (floor(x/y)=w728:T6)  [unwired: 1 out]
                  n449 = call "IMAQ Overlay Rectangle"("Color"=w734, "Group"="roi", "Rectangle"=w728, "Image"=w736) -> ("Image Out"=w733:T4)  [unwired: 6 in, 1 out]
                }
              }
            }
            n450 = local write "img_OD"(w713) -> ()
          }
        }
      }
      event "frame": Value Change {
        # "RAW DATA"
        # "redraw ROIs"
        # "Manually rescale to an I16"
        # "We've changed type, so switch color schemes"
        # "Do we actually have the frame we're supposed to show?"
        n451 = event-data() -> ("NewVal"=w756:i32, "OldVal"=w755:i32)  [unwired: 1 in]
        n452 = property on="image_data" class="Arr (strict)"() -> ("Value"=w759:u16[][][])  [unwired: 2 in, 2 out]
        n453 = Less Than 0?(x=w755) -> (x < 0?=w757:bool)
        n454 = Equal?(x=w756, y=w755) -> (x = y?=w753:bool)
        n455 = Array Size(array=w759) -> (size(s)=w752:i32[])
        n456 = Index Array(array=w752) -> (element=w751:i32)  [unwired: 1 in]
        n457 = Less?(x=w756, y=w751) -> (x < y?=w750:bool)
        n458 = Select(t=w756, s=w750, f=0) -> (s? t:f=w780:i32)
        n459 = Less Than 0?(x=w780) -> (x < 0?=w777:bool)
        n460 = local write "frame"(w780) -> ()
        n461 = Index Array(array=w759, index (dim 0)=w780) -> (element=w770:u16[][])  [unwired: 2 in]
        n462 = control-ref of="col_scheme"() -> (w779:refnum<vi>)
        n463 = control-ref of="raw_ctrls"() -> (w773:refnum<vi>)
        n464 = Exclusive Or(1:w757, 2:w777) -> (0:w778:bool)
        n465 = Or(x=w753, y=w778) -> (x .or. y?=w754:bool)
        n466 = case shown="True" w754 {
          tunnel: w779 -> [_ w784]
          frame False {
          }
          frame True {
            n467 = property class="Ring (strict)"(reference=w784) -> (reference out=w783:refnum<vi>, error out=w781:errorcluster, "Value"=w782:u16)  [unwired: 1 in]
            n468 = property class="Ring (strict)"(reference=w783, error in=w781, "Val(Sgnl)"=w782) -> ()  [unwired: 2 out]
          }
        }
        n469 = property class="Clust (strict)"(reference=w773) -> (reference out=w771:refnum<vi>, "Value"=w774:T30)  [unwired: 1 in, 1 out]
        n470 = Unbundle By Name(w774) -> ("automax"=w776:bool, "val_max"=w772:sgl, "val_min"=w775:sgl)
        n471 = Subtract(x=w770, y=w775) -> (x-y=w767:sgl[][])
        n472 = case shown="False" w776 {
          tunnel: [w785 w788] -> w763
          tunnel: w770 -> [_ w790]
          tunnel: w771 -> [_ w789]
          tunnel: w772 -> [w785 _]
          tunnel: w774 -> [_ w786]
          frame False {
          }
          frame True {
            # "Recompute maximum value"
            n473 = Array Max & Min(array=w790) -> (max value=w788:u16)  [unwired: 3 out]
            n474 = Bundle By Name(cluster=w786, "val_max"=w788) -> (w787:T30)
            n475 = property class="Clust (strict)"(reference=w789, "Value"=w787) -> ()  [unwired: 1 in, 2 out]
          }
        }
        n476 = Subtract(x=w763, y=w775) -> (x-y=w764:sgl)
        n477 = Divide(x=sgl 32767.0, y=w764) -> (x/y=w766:sgl)
        n478 = Multiply(x=w767, y=w766) -> (x*y=w768:sgl[][])
        n479 = local read "img_OD"() -> (w760:T4)
        n480 = To Word Integer(number=w768) -> (16bit integer=w758:i16[][])
        n481 = local read "rois"() -> (w762:T7)
        n482 = call "IMAQ ArrayToImage"("Image Pixels (I16)"=w758, "Image"=w760) -> ("error out"=w761:errorcluster, "Image Out"=w769:T4)  [unwired: 8 in]
        n483 = local write "img_OD"(w769) -> ()
        n484 = property on="rois" class="Arr (strict)"(error in=w761, "Val(Sgnl)"=w762) -> ()  [unwired: 1 in, 2 out]
      }
    }
  }
  n485 = while {
    tunnel: w59 -> [w800]
    tunnel: w29 -> [w793]
    tunnel: w60 -> [w795]
    stop <- FALSE stop-if-true
    # "Wait for TCP"
    # "Run forever"
    n486 = TCP Wait On Listener(11:w800) -> (0:w797:errorcluster, 1:w798:u16, 2:w799:string, 4:w794:refnum<k5>)  [unwired: 3 in, 1 out]
    n487 = Format Into String(format string=":%d", initial string=w799, w798) -> (resulting string=w801:string)  [unwired: 1 in, 1 out]
    n488 = Get Queue Status(queue=w795) -> (queue out=w792:refnum<queue>, queue name=w791:string)  [unwired: 2 in, 6 out]
    n489 = case shown="No Error" w797 {
      selector: w797 -> [_ w901]
      tunnel: w794 -> [w826 _]
      tunnel: w801 -> [w821 _]
      tunnel: w792 -> [w807 _]
      tunnel: w793 -> [w806 _]
      tunnel: w791 -> [w804 _]
      tunnel: w791 -> [w803 _]
      frame No Error {
        # "Receive data"
        n490 = TCP Read(connection ID=w826, bytes to read=1024, 7:T31."CRLF" ("mode (standard)"), 9:500 ("timeout ms (25000)")) -> (connection ID out=w818:refnum<k5>, data out=w823:string, error out=w820:errorcluster)  [unwired: 1 in]
        n491 = call <vilib>:"Trim Whitespace.vi"("string"=w823) -> ("trimmed string"=w822:string)  [unwired: 1 in]
        n492 = case shown="Default" w822 {
          selector: w822 -> [w864 _ _ _ _]
          tunnel: w821 -> [w863 _ _ _ _]
          tunnel: w820 -> [w858 _ _ _ _]
          tunnel: [_ "done\r\n" ("data in") w893 "hello\r\n" ("data in") _] -> w810
          tunnel: w807 -> [w860 w892 _ _ w899]
          tunnel: w806 -> [w859 w891 _ _ _]
          tunnel: [w855 w889 _ _ _] -> w808
          tunnel: w803 -> [w848 _ _ _ _]
          frame Default {
            w849 = errorcluster {"status"=FALSE, "code"=0, "source"=""} ("error in (no error)")
            # "check it's an HDF"
            n493 = Get Date/Time In Seconds() -> (seconds since 1Jan1904=w862:timestamp)
            n494 = String To Path(string=w864) -> (path=w856:path)
            n495 = Obtain Notifier(name (unnamed)=w848, notification data type=w849, error in (no error)=w849) -> (notifier out=w851:refnum<notifier>, error out=w853:errorcluster)  [unwired: 1 in, 1 out]
            n496 = Cancel Notification(0:w851, 3:w853) -> (8:w850:refnum<notifier>, 9:w854:errorcluster, 11:w852:errorcluster)
            n497 = Format Into String(format string="Received \"%s\" from %s at %T", w864, w863, w862) -> (resulting string=w861:string)  [unwired: 2 in, 1 out]
            n498 = call <vilib>:"H5F_is_hdf.vi"("error in (no error)"=w858, "path"=w856) -> ("valid"=w857:bool)  [unwired: 1 in, 2 out]
            n499 = Release Notifier(notifier=w850, error in (no error)=w852) -> ()  [unwired: 1 in, 3 out]
            n500 = call <userlib>:"BasicLogger.vi"("text"=w861) -> ()  [unwired: 6 in, 2 out]
            n501 = call <vilib>:"Clear Errors.vi"("error in (no error)"=w854) -> ()  [unwired: 6 in, 1 out]
            n502 = case shown="False" w857 {
              tunnel: w856 -> [w868 w881]
              tunnel: w860 -> [_ w883]
              tunnel: [w870 w873] -> w855
              tunnel: w859 -> [_ w882]
              frame False {
                n503 = Format Into String(format string="Received file \"%s\" not a valid HDF ", w868) -> (resulting string=w867:string)  [unwired: 2 in, 1 out]
                n504 = call <vilib>:"Error Cluster From Error Code.vi"("error message (\"\")"=w867, "error code (0)"=6042 ("t")) -> ("error out"=w870:errorcluster)  [unwired: 7 in]
              }
              frame True {
                n505 = call-dynamic "CameraAbort.vi"("CameraBase in"=w882) -> ("error out"=w872:errorcluster)  [unwired: 9 in, 1 out]
                n506 = call <vilib>:"Clear Errors.vi"("error in (no error)"=w872) -> ("error out"=w871:errorcluster)  [unwired: 6 in]
                n507 = Flush Queue(queue=w883, error in (no error)=w871) -> (queue out=w879:refnum<queue>, error out=w880:errorcluster)  [unwired: 1 out]
                n508 = flat-sequence {
                  tunnel: w881 -> [w884]
                  tunnel: w880 -> [w885]
                  tunnel: [w885] -> w875
                  frame #0 {
                    n509 = Strip Path(path=w884) -> (stripped path=w887:path, name=w886:string)
                    n510 = local write "working dir"(w887) -> ()
                    n511 = local write "current file"(w886) -> ()
                  }
                }
                n512 = Enqueue Element(queue=w879, element=Imaging_State."Read File", error in (no error)=w875) -> (queue out=w877:refnum<queue>, error out=w874:errorcluster)  [unwired: 1 in, 1 out]
                n513 = Enqueue Element(queue=w877, element=Imaging_State."Acquire", error in (no error)=w874) -> (error out=w873:errorcluster)  [unwired: 1 in, 2 out]
              }
            }
          }
          frame "abort" {
            # "BLACS signals abort"
            # "Kill the queue"
            # "Abort the camera"
            n514 = call-dynamic "CameraAbort.vi"("CameraBase in"=w891) -> ("error out"=w889:errorcluster)  [unwired: 9 in, 1 out]
            n515 = call <vilib>:"Clear Errors.vi"("error in (no error)"=w889) -> ("error out"=w890:errorcluster)  [unwired: 6 in]
            n516 = Flush Queue(queue=w892, error in (no error)=w890) -> ()  [unwired: 3 out]
          }
          frame "state" {
            n517 = local read "state"() -> (w895:T9)
            n518 = Format Into String(format string="%s\\r\\n", w895) -> (resulting string=w893:string)  [unwired: 2 in, 1 out]
          }
          frame "hello" {
            n519 = call <userlib>:"BasicLogger.vi"("text"="Received TCP ping") -> ()  [unwired: 6 in, 2 out]
          }
          frame "done" {
            n520 = Enqueue Element(queue=w899, element=Imaging_State."Save File") -> ()  [unwired: 2 in, 3 out]
            n521 = call <userlib>:"BasicLogger.vi"("text"="Received \"done\" command") -> ()  [unwired: 6 in, 2 out]
          }
        }
        n522 = case shown="\"\"" w810 {
          selector: w810 -> [w837 _]
          tunnel: w818 -> [w838 w845]
          tunnel: [w838 w842] -> w814
          tunnel: [w837 "done\r\n"] -> w813
          tunnel: [_ w841] -> w809
          tunnel: w808 -> [_ w840]
          tunnel: w804 -> [_ w839]
          frame Default {
          }
          frame "" {
            # "Make sure it worked"
            # "Send acknowledge response"
            n523 = TCP Write(connection ID=w845, data in="ok\r\n", 9:500 ("timeout ms (25000)")) -> (connection ID out=w842:refnum<k5>, error out=w847:errorcluster)  [unwired: 1 in, 1 out]
            n524 = call <vilib>:"Clear Errors.vi"("error in (no error)"=w847) -> ()  [unwired: 6 in, 1 out]
            n525 = call <userlib>:"Get_Notifier.vi"("error in"=w840, "name"=w839) -> ("error out"=w841:errorcluster)  [unwired: 1 in]
          }
        }
        n526 = case shown="No Error" w809 {
          selector: w809 -> [w832 _]
          tunnel: [w830 w836] -> w817
          tunnel: w813 -> [_ w836]
          tunnel: w807 -> [w828 _]
          tunnel: [w827 _] -> _
          tunnel: w806 -> [_ _]
          tunnel: [_ TRUE] -> w805
          frame Error {
            w831 = T14 0 items=["no dialog", "OK message", "continue or stop message", "OK message + warnings", "continue/stop + warnings"] ("type of dialog (OK msg:1)")
            # "Kill an acquisition if running (?)"
            # "kill any commands in the queue"
            # "Check if any errors occurred\nIf they did, BLACS will want to know"
            n527 = Flush Queue(queue=w828) -> ()  [unwired: 1 in, 3 out]
            n528 = call <vilib>:"Clear Errors.vi"() -> ()  [unwired: 7 in, 1 out]
            n529 = call <vilib>:"Simple Error Handler.vi"("type of dialog (OK msg:1)"=w831, "error in (no error)"=w832) -> ("error out"=w829:errorcluster, "message"=w833:string)  [unwired: 3 in, 3 out]
            n530 = Concatenate Strings("ERROR: " ("string"), w833) -> (w830:string)
            n531 = call <userlib>:"BasicErrorLogger.vi"("error in"=w829) -> ("error out"=w827:errorcluster)  [unwired: 1 in, 1 out]
          }
          frame No Error {
          }
        }
        n532 = TCP Write(connection ID=w814, data in=w817, 9:500 ("timeout ms (25000)")) -> (connection ID out=w812:refnum<k5>, error out=w815:errorcluster)  [unwired: 1 in, 1 out]
        n533 = local write "remote"(w805) -> ()
        n534 = TCP Close Connection(connection ID=w812, error in (no error)=w815) -> (error out=w819:errorcluster)  [unwired: 1 in, 1 out]
        n535 = call <vilib>:"Clear Errors.vi"("error in (no error)"=w819) -> ()  [unwired: 6 in, 1 out]
      }
      frame Error {
        n536 = call <userlib>:"BasicErrorLogger.vi"("error in"=w901) -> ()  [unwired: 1 in, 2 out]
      }
    }
  }
  n537 = Stop(stop? (T)=w62) -> ()
  "acquiring" <- w33
